vi "FEMC_TCP.vi"() -> ()   [LabVIEW 2017]
panel:
  in  "i-vクラスタ 2":T1={"start(mV)"=-1.0, "stop(mV)"=1.0, "step(mV)"=0.1, "file_name"="", "IF OFF/ON"=FALSE, "SAVE OFF/ON"=FALSE, "frq(GHz)"=8.0, "avg"=1, "Sweep回数 "=0, "VminfromSS"=0.15, "測定モード"=0, "V　opt"=2} {"測定モード" items=["電圧スイープ", "毎回HOT/COLD"]; "Sweep回数" items=["一回のみ", "Hot/Cold_auto", "Hot/Cold manual"]}
  out "GET_SIS_C 2":dbl=14.5172119140625
  out "GET_SIS_V 2":dbl=1.92230224609375
  in  "Control":T2={"GPIB_ATT"="28", "6501Dev#"=1, "GPIB_SP"="18", "GPIB_PM"="13", "GPIB_DSA"="11", "GPIB_DMM (TPD)"="23", "MPI COM"="COM5", "mortor設定"=[{"Axis"=0, "ID"=0, "HIspeed"=200.0, "LOspeed"=100.0, "ACCEL(ms)"=100.0, "Sratio"=50.0, "フリーラン\n"=FALSE, "文字列"="DSB HOT/COLD"}, {"Axis"=1, "ID"=0, "HIspeed"=4.0, "LOspeed"=4.0, "ACCEL(ms)"=100.0, "Sratio"=50.0, "フリーラン\n"=TRUE, "文字列"="SubMM Att"}, {"Axis"=0, "ID"=0, "HIspeed"=200.0, "LOspeed"=100.0, "ACCEL(ms)"=100.0, "Sratio"=50.0, "フリーラン\n"=FALSE, "文字列"="MPI Port1"}, {"Axis"=1, "ID"=0, "HIspeed"=200.0, "LOspeed"=100.0, "ACCEL(ms)"=100.0, "Sratio"=50.0, "フリーラン\n"=FALSE, "文字列"="MPI Port2"}, {"Axis"=1, "ID"=0, "HIspeed"=200.0, "LOspeed"=100.0, "ACCEL(ms)"=100.0, "Sratio"=50.0, "フリーラン\n"=TRUE, "文字列"="gainComp"}], "DATAパス"=path "C:/data/バランスドミクサ/150115/WCA_setmix_2", "mixer param file "=path "C:/data/バランスドミクサ/150115/mixparam_150115_balanced_Tmin_VSS1p5.csv", "comment"="150115_balanced_WCA_2", "Carteidge SN"="balanced150115", "Th"=297.0, "Tc"=83.26, "Set_SIS_volt"=2.1, "Offset"=0.0, "control"=0, "FreqLO"=799.0, "Set_Mag_Cur"=0.0, "MPI offset(mm)"=23.203, "HOT/COLD"=0} {"HOT/COLD" items=["DSB", "SBR (Cart.)"]; "control" items=["CLOSE LOOP", "OPEN LOOP", "Not Control"]}
  in  "i-vクラスタ":T1={"start(mV)"=-1.0, "stop(mV)"=1.0, "step(mV)"=0.1, "file_name"="", "IF OFF/ON"=FALSE, "SAVE OFF/ON"=FALSE, "frq(GHz)"=8.0, "avg"=1, "Sweep回数 "=0, "VminfromSS"=0.15, "測定モード"=0, "V　opt"=2} {"測定モード" items=["電圧スイープ", "毎回HOT/COLD"]; "Sweep回数" items=["一回のみ", "Hot/Cold_auto", "Hot/Cold manual"]}
  in  "demag":T3={"Start(mA)"=100.0, "Time(ms)"=200.0, "step"=1.0}
  in  "読み取りタイムアウト":i32=100
  in  "読み取りバイト数":i32=512
  in  "接続入力待ち（ms）":i32=10000
  out "接続回数":i32
  out "リモートポート":i16
  out "リモートアドレス":string
  out "接続中":bool
  out "GET_AMC":T4={"AMC_A_DRAIN_V"=3.5023499, "AMC_A_DRAIN_C"=53.95508, "AMC_A_GATE_V"=-0.47195435, "AMC_B_DRAIN_V"=4.3559265, "AMC_B_DRAIN_C"=314.81934, "AMC_B_GATE_V"=-0.49163818, "AMC_E_DRAIN_V"=3.9920044, "AMC_E_DRAIN_C"=338.2721, "AMC_E_GATE_V"=-0.24505615, "AMC_3V_SUPPLY_V"=-13.493347, "AMC_5V_MON"=5.223694, "AMC_MULT_D_V"=0.0}
  out "GET_PLL":T5={"PLL_ASSY_T"=35.217285, "PLL_REF_TOT_P"=-2.1250916, "PLL_IF_TOT_P"=-4.8457336, "PLL_CORR_V"=-0.14390425, "PLL_LOCK_V"=5.097532, "PLL_5V_SUPPLY_V"=18.560791, "Temp_TF"=TRUE, "PLL Ref Pwr_TF"=TRUE, "IF Pwr_TF"=TRUE, "PLL Corr_TF"=TRUE, "PLL Lock V_TF"=TRUE, "PLL Nominal_TF"=TRUE}
  out "GET_PA":T6={"PA_A_DRAIN_V"=2.3698425, "PA_A_DRAIN_C"=178.28369, "PA_A_GATE_V"=-0.3868103, "PA_B_DRAIN_V"=0.010070801, "PA_B_DRAIN_C"=5.996704, "PA_B_GATE_V"=-0.390625, "PA_3V_SUPPLY_V"=2.991333, "PA_5V_MON"=5.23407}
  out "SET_PA_VG":dbl
  out "SET_PA_VD":dbl
  out "GET_SIS_C":dbl=14.5172119140625
  out "GET_SIS_V":dbl=1.92230224609375
  out "SET_SIS_V":dbl=2.0
  in  "CLNA_SET":T7={"CLNA State"=1, "SET POL0 LNA1 STAGE1 DRAIN V"=1.2, "SET POL0 LNA1 STAGE1 DRAIN C"=14.0, "SET POL0 LNA1 STAGE2 DRAIN V"=0.0, "SET POL0 LNA1 STAGE2 DRAIN C"=0.0, "SET POL0 LNA1 STAGE3 DRAIN V"=0.0, "SET POL0 LNA1 STAGE3 DRAIN C"=0.0} {"SET POL0 LNA1 STAGE3 DRAIN C" min=0 max=20 step=0.01 format="%.2f"; "SET POL0 LNA1 STAGE3 DRAIN V" min=0 max=3 step=0.01 format="%.2f"; "SET POL0 LNA1 STAGE2 DRAIN C" min=0 max=20 step=0.01 format="%.2f"; "SET POL0 LNA1 STAGE2 DRAIN V" min=0 max=3 step=0.01 format="%.2f"; "SET POL0 LNA1 STAGE1 DRAIN C" min=0 max=20 step=0.01 format="%.2f"; "SET POL0 LNA1 STAGE1 DRAIN V" min=0 max=3 step=0.01 format="%.2f"; "CLNA State" items=["Disabled", "Enabled"]}
  out "CLNA_monitor":T8={"Pol0 LNA1 S1 Drain V [V]"=1.2019653, "Pol0 LNA1 S1 Drain C [mA]"=14.073029, "Pol0 LNA1 S1 Gate V [V]"=0.5575104, "Pol0 LNA1 S2 Drain V [V]"=0.0029144287, "Pol0 LNA1 S2 Drain C [mA]"=0.00076293945, "Pol0 LNA1 S2 Gate V [V]"=4.940506, "Pol0 LNA1 S3 Drain V [V]"=0.0027313232, "Pol0 LNA1 S3 Drain C [mA]"=0.025024414, "Pol0 LNA1 S3 Gate V [V]"=4.9404755, "Pol0 LNA1 State"=enum."Enabled"} {"Pol0 LNA1 S3 Gate V [V]" format="%.2f"; "Pol0 LNA1 S3 Drain C [mA]" format="%.2f"; "Pol0 LNA1 S3 Drain V [V]" format="%.2f"; "Pol0 LNA1 S2 Gate V [V]" format="%.2f"; "Pol0 LNA1 S2 Drain C [mA]" format="%.2f"; "Pol0 LNA1 S2 Drain V [V]" format="%.2f"; "Pol0 LNA1 S1 Gate V [V]" format="%.2f"; "Pol0 LNA1 S1 Drain C [mA]" format="%.2f"; "Pol0 LNA1 S1 Drain V [V]" format="%.2f"}
  in  "SIScontrol":u16(ring) items=["CLOSE LOOP", "OPEN LOOP", "Not Control"]
  out "option":string
  in  "Bias_LO_equip":T9={"Node address"=19, "CAN Interface"="CAN0", "Cartridge band"=8, "Slave Node in"={"Address"=19, "Serial Number"=[16, 121, 69, 76, 1, 8, 0, -31]}, "ObjHandle out"=20, "POL"=0, "sb"=1, "GPIB_SM (SIS S,V)"="24", "GPIB_DMM (SIS I)"="22", "GPIB_SM (MAG I) "="25", "GPIB_SG(LO)"="19", "GPIB_PW (PAMP) "="6", "GPIB_TMP1(8ch)"="12", "GPIB_TMP2(2ch)  "="13", "WCA_avg"=10, "Rsen"=10.0, "BiasModule"=1, "LOModule "=2, "WCA_LO_FREQ_SET"={"YTO Low freq. [GHz]"=14.65, "YTO High freq. [GHz]"=17.5, "Kvco"=1, "Lock Pol."=0, "SET LO FREQ"=88.77778, "Multiplier"=6.0, "YTO (HEX)"=210, "YTO ( FREQ)"=14.796153, "NULL PLL INTEGRATOR"=TRUE}, "Res for"=0} {"Res for" items=["none", "series res", "parallel res"]; "WCA_LO_FREQ_SET"."YTO ( FREQ)" min=25 max=150 step=0.0001 format="%.3f"; "WCA_LO_FREQ_SET"."Multiplier" min=3 max=6 step=3; "WCA_LO_FREQ_SET"."SET LO FREQ" min=25 max=150 step=0.0001 format="%.3f"; "WCA_LO_FREQ_SET"."Lock Pol." items=["Lower", "Upper"]; "WCA_LO_FREQ_SET"."Kvco" items=["7.5MHz/V", "15MHz/V"]; "WCA_LO_FREQ_SET"."YTO High freq. [GHz]" format="%.3f"; "WCA_LO_FREQ_SET"."YTO Low freq. [GHz]" format="%.3f"; "BiasModule" items=["B10Lab Bias"=0, "WCA BiasModule"=1, "none"=99]; "Slave Node in"."Serial Number" format="%.0x"; "Slave Node in"."Address" format="%.0x"; "Cartridge band" max=10 step=1; "Node address" format="%.0x"}
  out "send message":string
  in  "exit":bool=TRUE caption="停止"
  in  "stop":bool caption="停止"
  out "command:":string caption="command"
  out "c ID":refnum<k5> caption="接続ID"
  in  "Port":u16=7568 caption="サーバーポート"
  # "Vd [V]"
  # "Id [mA]"
  # "Vg [V]"
  # "AMC A"
  # "AMC B"
  # "AMC E"
  # "-3V/5V Supply"
  # "Vd [V]"
  # "Id [mA]"
  # "Vg [V]"
  # "PA A"
  # "PA B"
  # "Vd [V]"
  # "Id [mA]"
  # "Stage 1"
  # "Stage 2"
  # "Stage 3"
  # "CLNA State."
  # "Vd [V]"
  # "Id [mA]"
  # "Vg [V]"
  # "Stage 1"
  # "Stage 2"
  # "Stage 3"
  # "LO freq. [GHz]"
  # "YTO LOW\n/High Freq."
  # "ZERO Intgrtr"
  # "Node Address"
  # "Serial Number"
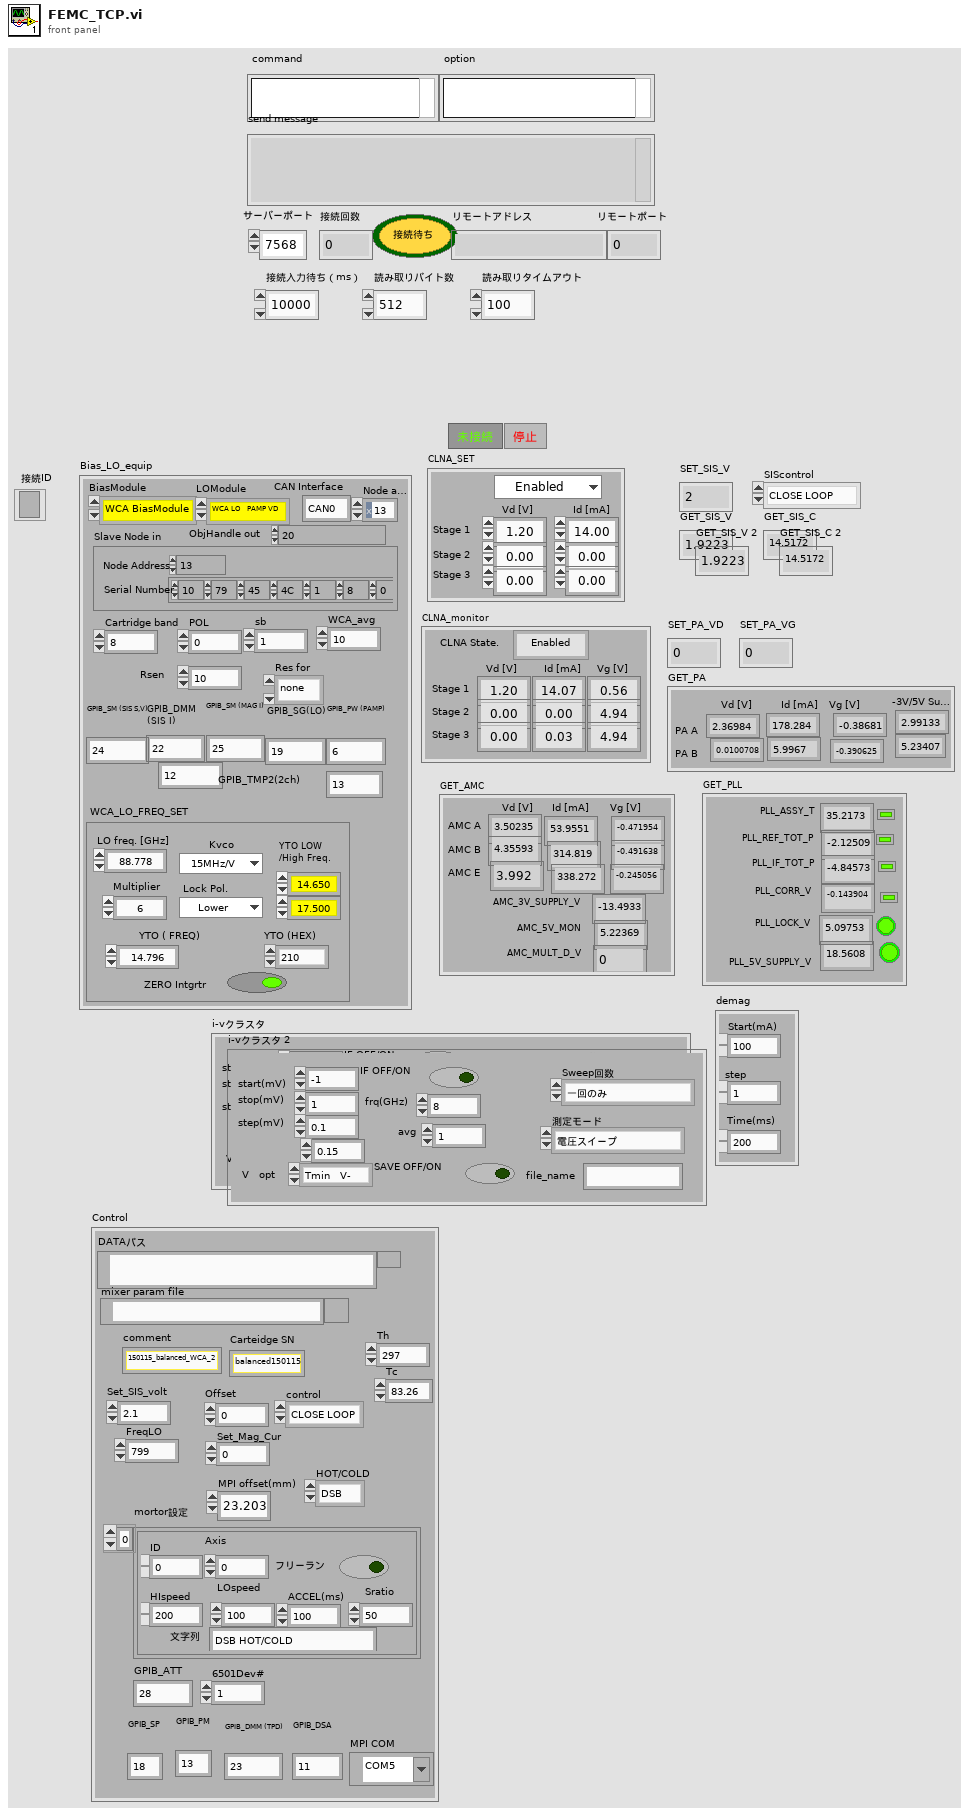
[diagram p1: front panel]
types:
  T1 = cluster{"start(mV)":dbl, "stop(mV)":dbl, "step(mV)":dbl, "file_name":string, "IF OFF/ON":bool, "SAVE OFF/ON":bool, "frq(GHz)":dbl, "avg":i32, "Sweep回数 ":u16, "VminfromSS":dbl, "測定モード":u16, "V　opt":u16}
  T2 = cluster{"GPIB_ATT":string, "6501Dev#":i16, "GPIB_SP":string, "GPIB_PM":string, "GPIB_DSA":string, "GPIB_DMM (TPD)":string, "MPI COM":refnum<visa-resource-name>, "mortor設定":cluster{"Axis":i16, "ID":i16, "HIspeed":dbl, "LOspeed":dbl, "ACCEL(ms)":dbl, "Sratio":dbl, "フリーラン\n":bool, "文字列":string}[], "DATAパス":path, "mixer param file ":path, "comment":string, "Carteidge SN":string, "Th":dbl, "Tc":dbl, "Set_SIS_volt":dbl, "Offset":dbl, "control":u16, "FreqLO":dbl, "Set_Mag_Cur":dbl, "MPI offset(mm)":dbl, "HOT/COLD":u16}
  T3 = cluster{"Start(mA)":dbl, "Time(ms)":dbl, "step":dbl}
  T4 = cluster{"AMC_A_DRAIN_V":sgl, "AMC_A_DRAIN_C":sgl, "AMC_A_GATE_V":sgl, "AMC_B_DRAIN_V":sgl, "AMC_B_DRAIN_C":sgl, "AMC_B_GATE_V":sgl, "AMC_E_DRAIN_V":sgl, "AMC_E_DRAIN_C":sgl, "AMC_E_GATE_V":sgl, "AMC_3V_SUPPLY_V":sgl, "AMC_5V_MON":sgl, "AMC_MULT_D_V":sgl}
  T5 = cluster{"PLL_ASSY_T":sgl, "PLL_REF_TOT_P":sgl, "PLL_IF_TOT_P":sgl, "PLL_CORR_V":sgl, "PLL_LOCK_V":sgl, "PLL_5V_SUPPLY_V":sgl, "Temp_TF":bool, "PLL Ref Pwr_TF":bool, "IF Pwr_TF":bool, "PLL Corr_TF":bool, "PLL Lock V_TF":bool, "PLL Nominal_TF":bool}
  T6 = cluster{"PA_A_DRAIN_V":sgl, "PA_A_DRAIN_C":sgl, "PA_A_GATE_V":sgl, "PA_B_DRAIN_V":sgl, "PA_B_DRAIN_C":sgl, "PA_B_GATE_V":sgl, "PA_3V_SUPPLY_V":sgl, "PA_5V_MON":sgl}
  T7 = cluster{"CLNA State":u8, "SET POL0 LNA1 STAGE1 DRAIN V":sgl, "SET POL0 LNA1 STAGE1 DRAIN C":sgl, "SET POL0 LNA1 STAGE2 DRAIN V":sgl, "SET POL0 LNA1 STAGE2 DRAIN C":sgl, "SET POL0 LNA1 STAGE3 DRAIN V":sgl, "SET POL0 LNA1 STAGE3 DRAIN C":sgl}
  T8 = cluster{"Pol0 LNA1 S1 Drain V [V]":sgl, "Pol0 LNA1 S1 Drain C [mA]":sgl, "Pol0 LNA1 S1 Gate V [V]":sgl, "Pol0 LNA1 S2 Drain V [V]":sgl, "Pol0 LNA1 S2 Drain C [mA]":sgl, "Pol0 LNA1 S2 Gate V [V]":sgl, "Pol0 LNA1 S3 Drain V [V]":sgl, "Pol0 LNA1 S3 Drain C [mA]":sgl, "Pol0 LNA1 S3 Gate V [V]":sgl, "Pol0 LNA1 State":enum16{"Disabled", "Enabled"}}
  T9 = cluster{"Node address":u16, "CAN Interface":string, "Cartridge band":u32, "Slave Node in":cluster{"Address":i16, "Serial Number":i8[]}, "ObjHandle out":u32, "POL":u32, "sb":u32, "GPIB_SM (SIS S,V)":string, "GPIB_DMM (SIS I)":string, "GPIB_SM (MAG I) ":string, "GPIB_SG(LO)":string, "GPIB_PW (PAMP) ":string, "GPIB_TMP1(8ch)":string, "GPIB_TMP2(2ch)  ":string, "WCA_avg":i32, "Rsen":dbl, "BiasModule":u16, "LOModule ":u16, "WCA_LO_FREQ_SET":cluster{"YTO Low freq. [GHz]":sgl, "YTO High freq. [GHz]":sgl, "Kvco":u16, "Lock Pol.":u16, "SET LO FREQ":sgl, "Multiplier":sgl, "YTO (HEX)":u16, "YTO ( FREQ)":sgl, "NULL PLL INTEGRATOR":bool}, "Res for":u16}
  T10 = cluster{"Node address":u16, "CAN Interface":string, "Cartridge band":u32, "Slave Node in":cluster{"Address":i16, "Serial Number":i8[]}, "ObjHandle out":u32, "POL":u32, "sb":u32, "GPIB_SM (SIS S,V)":string, "GPIB_DMM (SIS I)":string, "GPIB_SM (MAG I) ":string, "GPIB_SG(LO)":string, "GPIB_PW (PAMP) ":string, "GPIB_TMP1(8ch)":string, "GPIB_TMP2(2ch)  ":string, "WCA_avg":i32, "Rsen":dbl, "BiasModule":u16, "LOModule ":u16, "WCA_LO_FREQ_SET":cluster{"YTO Low freq. [GHz]":sgl, "YTO High freq. [GHz]":sgl, "Kvco":u16, "Lock Pol.":u16, "SET LO FREQ":sgl, "Multiplier":sgl, "YTO (HEX)":u16, "YTO coarse( FREQ)":sgl, "NULL PLL INTEGRATOR":bool}, "Res for":u16}
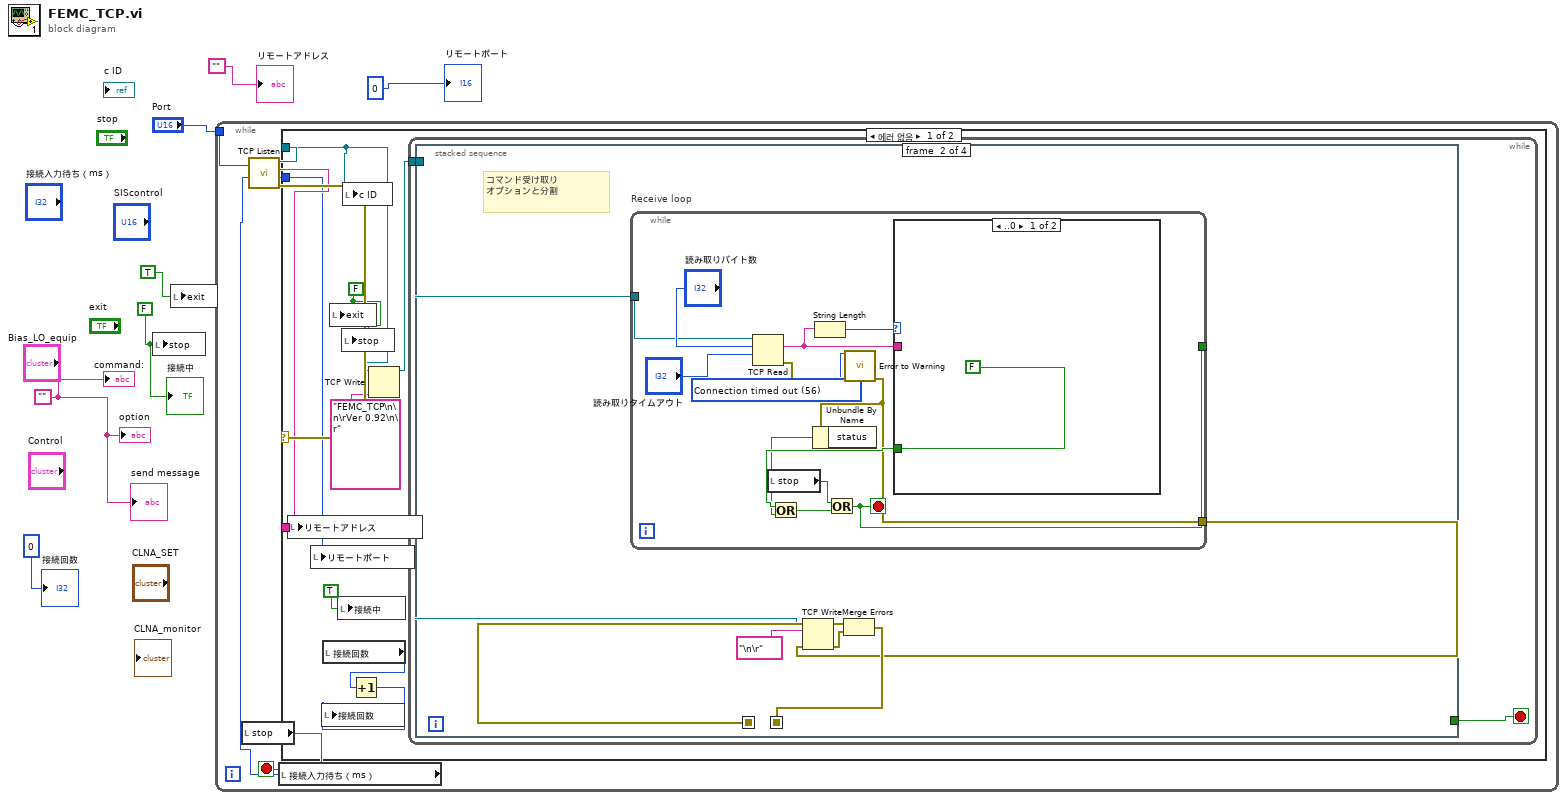
[diagram p0: block diagram]
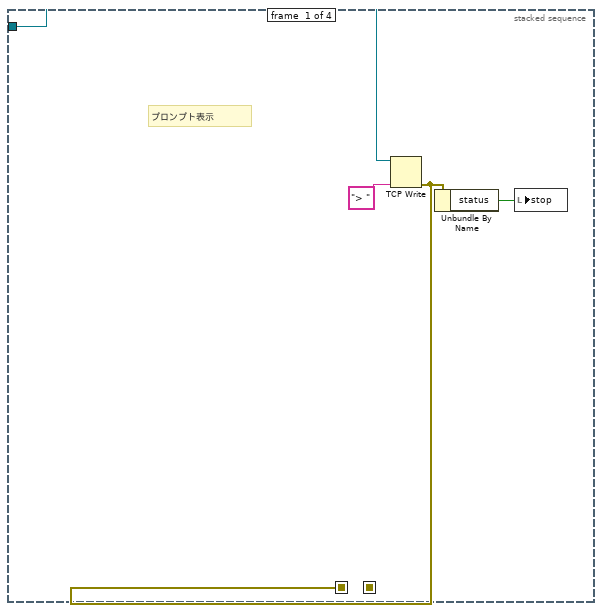
[diagram p2: hidden frame]
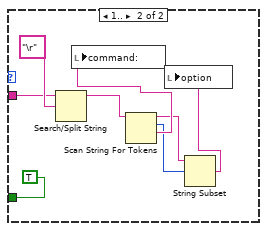
[diagram p3: hidden frame]
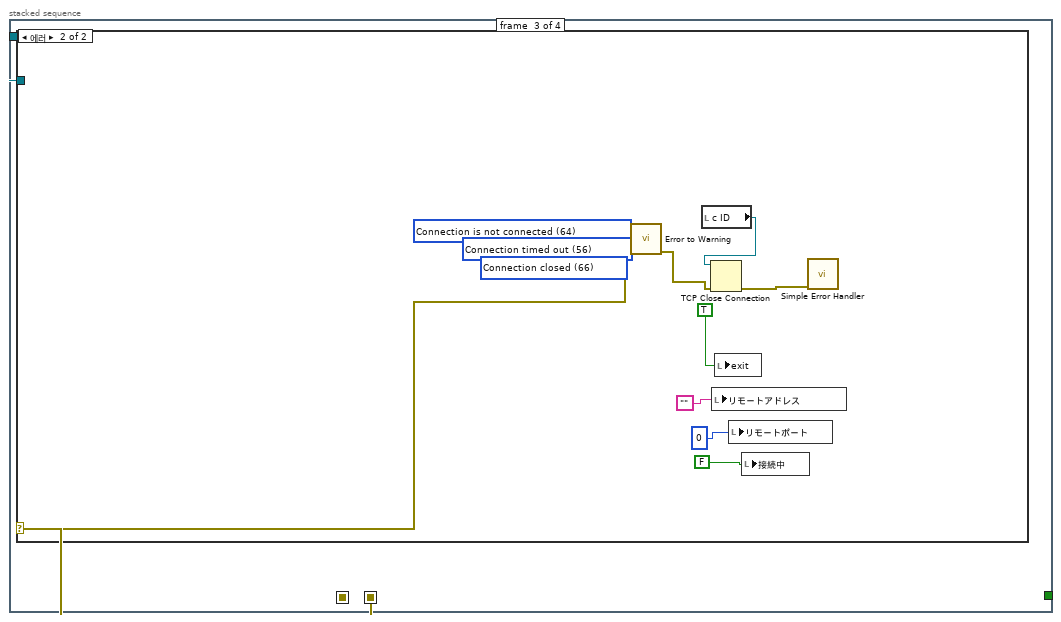
[diagram p4: hidden frame]
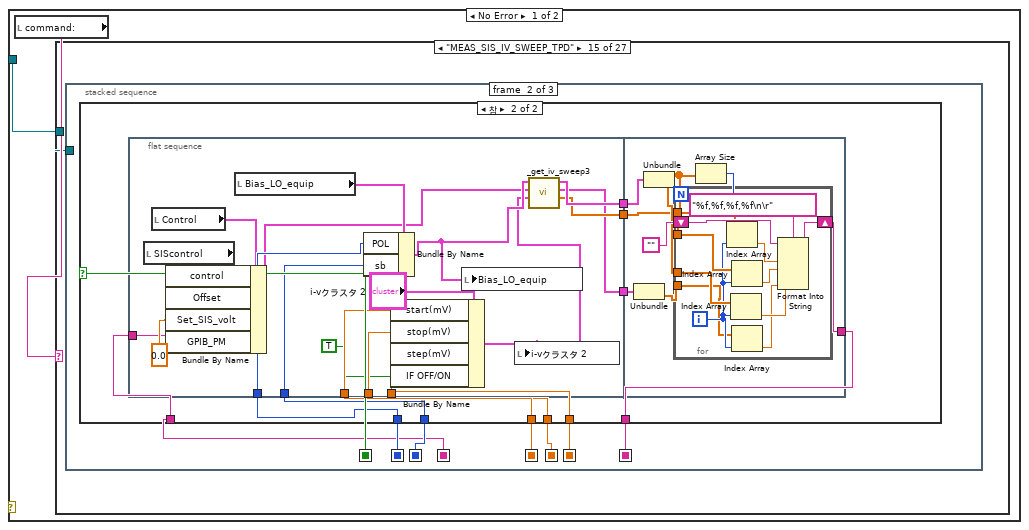
[diagram p5: hidden frame]
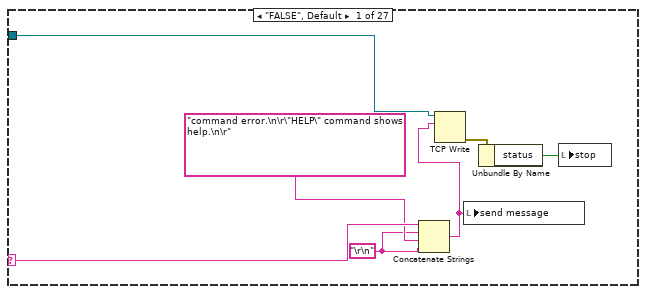
[diagram p6: hidden frame]
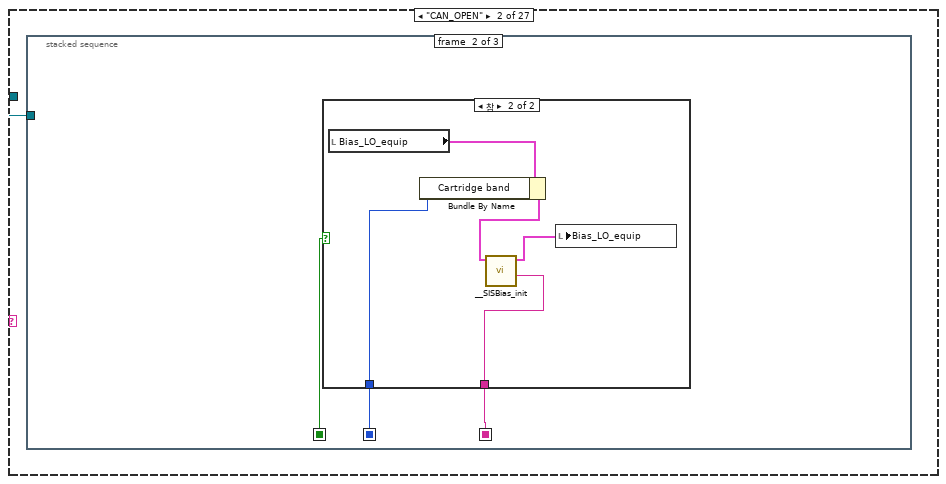
[diagram p7: hidden frame]
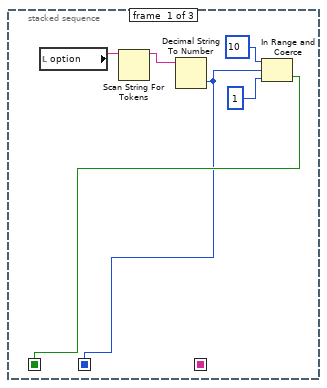
[diagram p8: hidden frame]
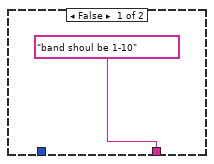
[diagram p9: hidden frame]
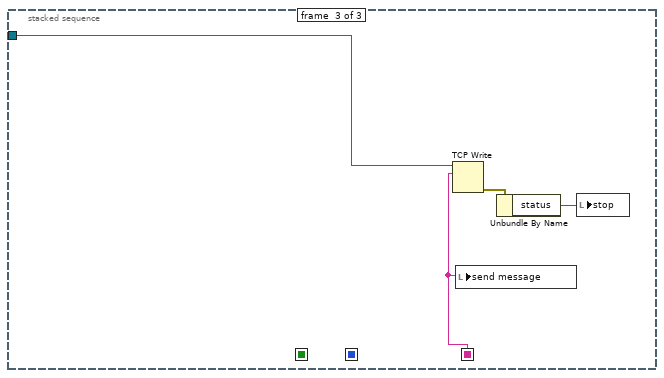
[diagram p10: hidden frame]
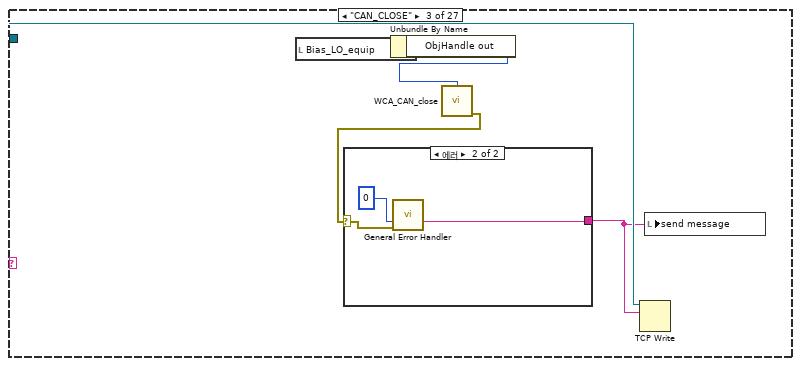
[diagram p11: hidden frame]
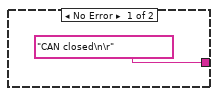
[diagram p12: hidden frame]
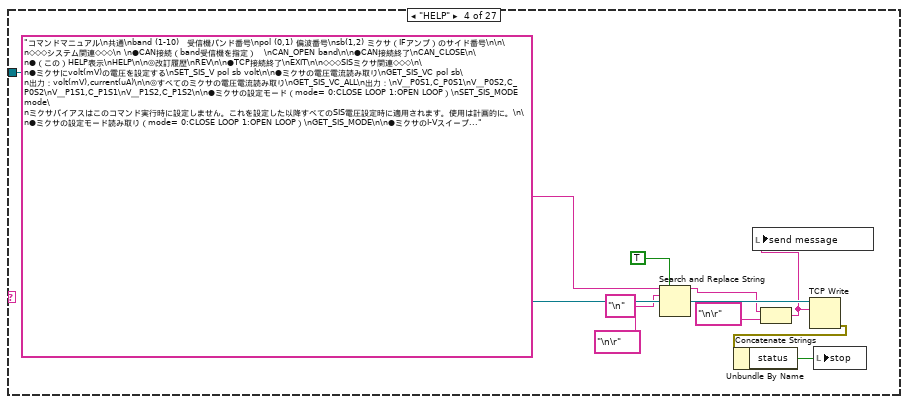
[diagram p13: hidden frame]
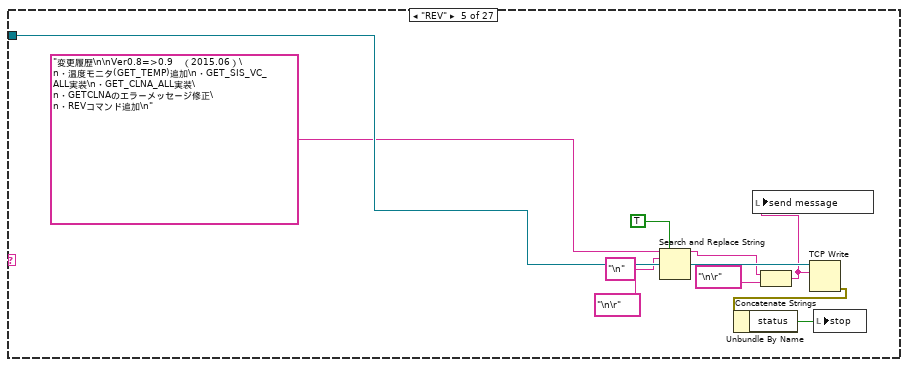
[diagram p14: hidden frame]
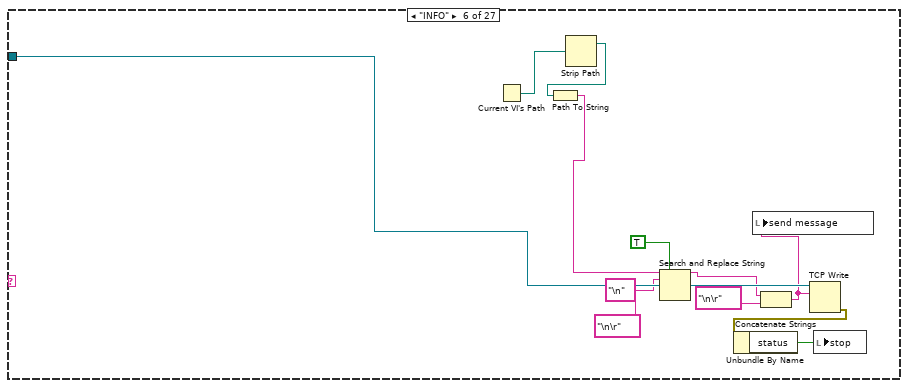
[diagram p15: hidden frame]
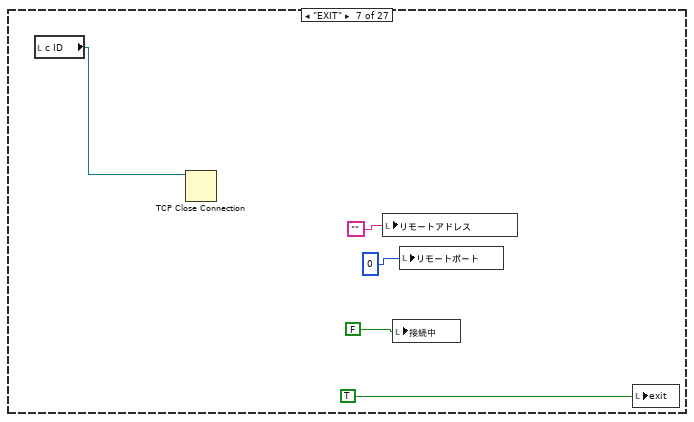
[diagram p16: hidden frame]
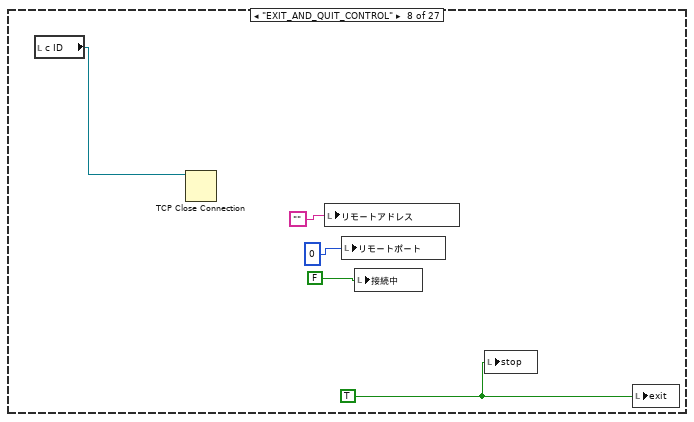
[diagram p17: hidden frame]
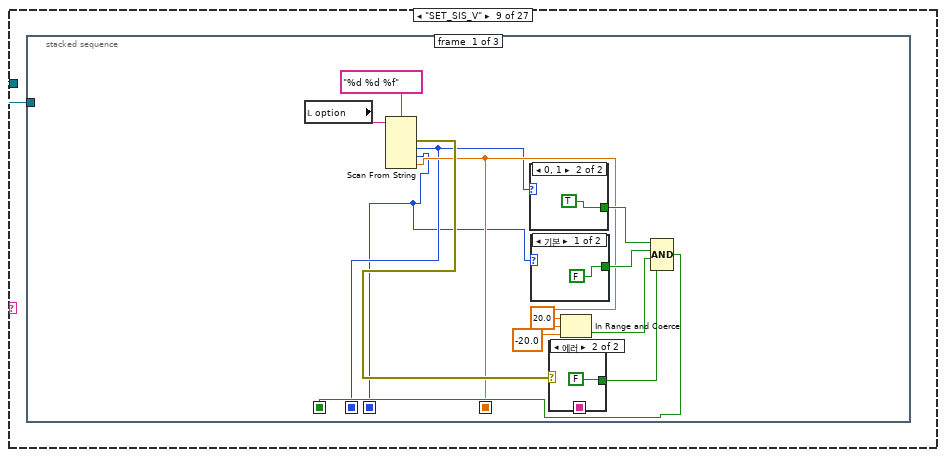
[diagram p18: hidden frame]
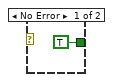
[diagram p19: hidden frame]
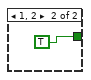
[diagram p20: hidden frame]
diagram:
  w1 = ""
  w5 = FALSE
  n1 = local write "stop"(w5) -> ()
  n2 = local write "exit"(TRUE) -> ()
  n3 = while {
    tunnel: "Port" -> [w14]
    stop <- w13 stop-if-true
    n4 = local read "stop"() -> (w13:bool)
    n5 = local read "接続入力待ち（ms）"() -> (w8:i32)
    n6 = call <vilib>:"TCP Listen.vi"("timeout ms (wait forever: -1)"=w8, "port"=w14) -> ("error out"=w12:errorcluster, "remote port"=w9:u16, "remote address"=w10:string, "connection ID"=w11:refnum<k5>)  [unwired: 5 in, 1 out]
    n7 = case shown="에러 없음" w12 {
      tunnel: w11 -> [w22 _]
      tunnel: w10 -> [w19 _]
      tunnel: w9 -> [w18 _]
      frame No Error {
        w20 = FALSE
        n8 = local write "リモートアドレス"(w19) -> ()
        n9 = local write "リモートポート"(w18) -> ()
        n10 = local read "接続回数"() -> (w16:i32)
        n11 = local write "exit"(w20) -> ()
        n12 = local write "接続中"(TRUE) -> ()
        n13 = local write "stop"(w20) -> ()
        n14 = local write "c ID"(w22) -> ()
        n15 = Increment(x=w16) -> (x+1=w15:i32)
        n16 = local write "接続回数"(w15) -> ()
        n17 = TCP Write(connection ID=w22, data in="FEMC_TCP\n\n\rVer 0.92\n\r") -> (connection ID out=w21:refnum<k5>)  [unwired: 2 in, 2 out]
        n18 = while {
          tunnel: w21 -> [w24]
          stop <- w25 stop-if-true
          n19 = stacked-sequence {
            seq-local: [w27 _ _ _] -> [_ w35 _ _]
            seq-local: [_ w34 _ _] -> [_ _ w59 _]
            tunnel: w24 -> [w29 w30 w58 _]
            tunnel: [_ _ _ w1048] -> w25
            frame #0 {
              # "プロンプト表示"
              n20 = TCP Write(connection ID=w29, data in="> ") -> (error out=w27:errorcluster)  [unwired: 2 in, 2 out]
              n21 = Unbundle By Name(w27) -> ("status"=w28:bool)
              n22 = local write "stop"(w28) -> ()
            }
            frame #1 {
              # "コマンド受け取り\nオプションと分割"
              n23 = while "Receive loop" {
                tunnel: [w45] -> _
                tunnel: [w39] -> w31
                tunnel: w30 -> [w46]
                stop <- w45 stop-if-true
                w40 = 56 items=["No Error", "Argument Error", "Memory Full", "Out of Zone", "End of File", "File Already Open", "Generic File IO Error", "File Not Found", "File Permission Error", "Disk Full", "Duplicate Path", "Too Many Files Open", "Not Enabled", "Resource File Not Found", "Cannot Add Resource", "Resource Not Found", "Image Not Found", "Image Memory Error", "Pen Does Not Exist", "Config Bad Type", "Config Token Not Found", "Config Parse Error", "Config Memory Error", "Bad External Code Format", "Bad External Code Offset", "External Code Not Present", "Null Window", "Destroy Window Mixup", "Null Menu", "Print Aborted", "Bad Print Record", "Print Driver Error", "Windows Error During Print", "Memory Error During Print", "Print Dialog Error", "Generic Print Error", "Invalid Device Refnum", "Device Not Found", "Device Parameter Error", "Device Unit Error", "Can't Open Device", "Device Call Aborted", "Generic Error", "Cancelled By User", "Object ID Too Low", "Object ID Too High", "Object Not In Heap", "Unknown Heap", "Bad DefProc ID", "DefProc Not In Table", "Message Out Of Range", "Null Method", "Unknown Message", "Manager Call Not Supported", "Bad address", "Connection In progress", "Connection timed out", "Connection is already in progress", "Network attribute not supported", "Network error", "Address in use", "System out of memory", "Connection aborted", "Connection refused", "Connection is not connected", "Connection is already connected", "Connection closed", "Initialize error (interapplication manager)", "Bad occurrence", "Wait on unbound occurrence handler", "Occurrence queue overflow", "Bad path", "Semaphore not signaled", "Unrecognized type (interapplication manager)"] ("1st Error to Convert")
                n24 = TCP Read(connection ID=w46, bytes to read="読み取りバイト数", 9:"読み取りタイムアウト") -> (data out=w44:string, error out=w41:errorcluster)  [unwired: 2 in, 1 out]
                n25 = local read "stop"() -> (w37:bool)
                n26 = String Length(string=w44) -> (length=w48:i32)
                n27 = call <vilib>:"Error to Warning.vi"("1st Error to Convert"=w40, "error in"=w41) -> ("warning out"=w39:errorcluster)  [unwired: 13 in]
                n28 = Unbundle By Name(w39) -> ("status"=w38:bool)
                n29 = case shown="..0" w48 {
                  tunnel: w44 -> [_ w55]
                  tunnel: [FALSE TRUE] -> w43
                  frame ..0 {
                  }
                  frame 1.. {
                    n30 = Search/Split String(string=w55, search string/char (-)="\r") -> (substring before match=w54:string)  [unwired: 1 in, 2 out]
                    n31 = Scan String For Tokens(9:w54) -> (1:w53:string, 2:w51:i32, 3:w52:string)  [unwired: 5 in, 1 out]
                    n32 = local write "command:"(w53) -> ()
                    n33 = String Subset(string=w52, offset (0)=w51) -> (substring=w50:string)  [unwired: 1 in]
                    n34 = local write "option"(w50) -> ()
                  }
                }
                n35 = Or(x=w43, y=w38) -> (x .or. y?=w36:bool)
                n36 = Or(x=w37, y=w36) -> (x .or. y?=w45:bool)
              }
              n37 = TCP Write(connection ID=w30, data in="\n\r", error in (no error)=w31) -> (error out=w32:errorcluster)  [unwired: 1 in, 2 out]
              n38 = Merge Errors(w35, w32) -> (w34:errorcluster)
            }
            frame #2 {
              n39 = case shown="에러" w59 {
                selector: w59 -> [_ w1041]
                tunnel: w58 -> [w61 _]
                frame No Error {
                  n40 = local read "command:"() -> (w60:string)
                  n41 = case shown="\"MEAS_SIS_IV_SWEEP_TPD\"" w60 {
                    selector: w60 -> [w65 _ _ _ _ _ _ _ _ _ _ _ _ _ _ _ _ _ _ _ _ _ _ _ _ _ _]
                    tunnel: w61 -> [w66 w69 w90 w105 w115 w127 _ _ w140 w183 w222 w250 w274 w283 w363 w454 w551 w605 w648 w691 w727 w760 w816 w858 w900 w950 w1009]
                    frame "FALSE", Default {
                      w63 = "\r\n"
                      n42 = Concatenate Strings(w65, w63, "command error.\n\r\"HELP\" command shows  help.\n\r", w63) -> (w62:string)
                      n43 = TCP Write(connection ID=w66, data in=w62) -> (error out=w67:errorcluster)  [unwired: 2 in, 2 out]
                      n44 = local write "send message"(w62) -> ()
                      n45 = Unbundle By Name(w67) -> ("status"=w68:bool)
                      n46 = local write "stop"(w68) -> ()
                    }
                    frame "CAN_OPEN" {
                      n47 = stacked-sequence {
                        seq-local: [w71 _ _] -> [_ w78 _]
                        seq-local: [w70 _ _] -> [_ w77 _]
                        seq-local: [_ w76 _] -> [_ _ w85]
                        tunnel: w69 -> [_ _ w86]
                        frame #0 {
                          n48 = local read "option"() -> (w75:string)
                          n49 = Scan String For Tokens(9:w75) -> (3:w74:string)  [unwired: 5 in, 3 out]
                          n50 = Decimal String To Number(string=w74) -> (number=w70:i32)  [unwired: 2 in, 1 out]
                          n51 = In Range and Coerce(upper limit=10, x=w70, lower limit=1) -> (In Range?=w71:bool)  [unwired: 1 out]
                        }
                        frame #1 {
                          n52 = case shown="참" w78 {
                            tunnel: w77 -> [_ w83]
                            tunnel: ["band shoul be 1-10" w80] -> w76
                            frame False {
                            }
                            frame True {
                              n53 = local read "Bias_LO_equip"() -> (w84:T9)
                              n54 = Bundle By Name(cluster=w84, "Cartridge band"=w83) -> (w82:T9)
                              n55 = call "__SISBias_init.vi"("Bias_LO_equip"=w82) -> ("Detected CAN Nodes."=w80:string, "Bias_LO_equip 2"=w81:T10)  [unwired: 4 in, 1 out]
                              n56 = local write "Bias_LO_equip"(w81) -> ()
                            }
                          }
                        }
                        frame #2 {
                          n57 = TCP Write(connection ID=w86, data in=w85) -> (error out=w87:errorcluster)  [unwired: 2 in, 2 out]
                          n58 = local write "send message"(w85) -> ()
                          n59 = Unbundle By Name(w87) -> ("status"=w88:bool)
                          n60 = local write "stop"(w88) -> ()
                        }
                      }
                    }
                    frame "CAN_CLOSE" {
                      n61 = local read "Bias_LO_equip"() -> (w93:T9)
                      n62 = Unbundle By Name(w93) -> ("ObjHandle out"=w92:u32)
                      n63 = call "WCA_CAN_close.vi"("ObjHandle in"=w92) -> ("error out"=w91:errorcluster)  [unwired: 14 in]
                      n64 = case shown="에러" w91 {
                        selector: w91 -> [_ w97]
                        tunnel: ["CAN closed\n\r" w96] -> w89
                        frame No Error {
                        }
                        frame Error {
                          n65 = call <vilib>:"General Error Handler.vi"("type of dialog (OK msg:1)"=0, "error in (no error)"=w97) -> ("message"=w96:string)  [unwired: 9 in, 4 out]
                        }
                      }
                      n66 = TCP Write(connection ID=w90, data in=w89) -> ()  [unwired: 2 in, 3 out]
                      n67 = local write "send message"(w89) -> ()
                    }
                    frame "HELP" {
                      n68 = Search and Replace String(replace all?=TRUE, input string="コマンドマニュアル\n共通\nband (1-10)　受信機バンド番号\npol (0,1) 偏波番号\nsb(1,2) ミクサ（IFアンプ）のサイド番号\n\n\n◇◇◇システム関連◇◇◇\n \n●CAN接続（band受信機を指定）　\nCAN_OPEN band\n\n●CAN接続終了\nCAN_CLOSE\n\n●（この）HELP表示\nHELP\n\n◎改訂履歴\nREV\n\n●TCP接続終了\nEXIT\n\n◇◇◇SISミクサ関連◇◇◇\n\n●ミクサにvolt(mV)の電圧を設定する\nSET_SIS_V pol sb volt\n\n●ミクサの電圧電流読み取り\nGET_SIS_VC pol sb\n出力：volt(mV),current(uA)\n\n◎すべてのミクサの電圧電流読み取り\nGET_SIS_VC_ALL\n出力：\nV＿P0S1,C_P0S1\nV＿P0S2,C_P0S2\nV＿P1S1,C_P1S1\nV＿P1S2,C_P1S2\n\n●ミクサの設定モード（mode= 0:CLOSE LOOP 1:OPEN LOOP）\nSET_SIS_MODE mode\nミクサバイアスはこのコマンド実行時に設定しません。これを設定した以降すべてのSIS電圧設定時に適用されます。使用は計画的に。\n\n●ミクサの設定モード読み取り（mode= 0:CLOSE LOOP 1:OPEN LOOP）\nGET_SIS_MODE\n\n●ミクサのI-Vスイープ\nMEAS_SIS_IV_SWEEP pol sb start stop step\n出力：v,iの連続データ\n\n●ミクサのI-VスイープWHSFのTPDからデータ取得\nMEAS_SIS_IV_SWEEP_TPD pol sb start stop step IP_TPDnum\n\nIP_TPD_num:TPD//IPアドレス//TPD番号（1から8）\n例：TPD//192.168.11.194//1\n出力：v,iの連続データ\n\n\n◇◇◇CLNA関連◇◇◇\n\n●CLNAにVD=vd#(V),ID=id#(mA)のバイアス設定(と同時に電源ONします)\nSET_CLNA pol sb vd1 id1 vd2 id2 vg3 id3\n\n●CLNAのバイアス読み取り\nGET_CLNA pol sb\n出力：vd1(V),id1(mA),vg1(V),vd2(V),id2(mA)vg2(V),vd3(V),id3(mA)vg3(V),ENABLED(1) or DISABLED(0)\n\n●CLNAの電源OFF\nSET_CLNA_OFF pol sb\n\n◎すべてのCLNAのバイアス読み取り\nGET_CLNA_ALL \n出力：\nP0S1:vd1(V),id1(mA),vg1(V),vd2(V),id2(mA)vg2(V),vd3(V),id3(mA)vg3(V),ENABLED(1) or DISABLED(0)\nP0S2:vd1(V),id1(mA),vg1(V),vd2(V),id2(mA)vg2(V),vd3(V),id3(mA)vg3(V),ENABLED(1) or DISABLED(0)\nP1S1:vd1(V),id1(mA),vg1(V),vd2(V),id2(mA)vg2(V),vd3(V),id3(mA)vg3(V),ENABLED(1) or DISABLED(0)\nP1S2:vd1(V),id1(mA),vg1(V),vd2(V),id2(mA)vg2(V),vd3(V),id3(mA)vg3(V),ENABLED(1) or DISABLED(0)\n\n\n\n◇◇◇超伝導コイル関連◇◇◇\n\n●超伝導コイル　current(mA)設定\nSET_MAG_C pol sb current\n\n●超伝導コイル電圧電流読み取り\nGET_MAG_VC pol sb(範囲確認)\n出力：volt(V),current(mA)\n\n●超伝導コイル　消磁（demag,deflux）\nACT_DEMAG pol sb start step time\nstart(mA)からstep(mA)毎にtime(ms)で0mAになるまでDemagを行う。\n実行時設定電流は以下の通り、\n+start, 0, -start, 0,\n+(start-step), 0,-(start-step)\n, , , \n0\n\n\n\n◇◇◇WCA-LO関連◇◇◇\n\n●LO PAMPのvd(V)設定（pol=0:PA-A 1:PA-B）\nSET_PA_VD pol vd(範囲確認)\n\n●LO PAMPのvg(V)設定（pol=0:PA-A 1:PA-B）\nSET_PA_VG pol vg(範囲確認)\n\n●LO PAMPのvd(V),vg(V)読み取り（pol=0:PA-A 1:PA-B）\nGET_PA pol\n出力：vd(V),id(mA),vg(V)\n\n●WCA_LOの電源等パラメータ読み取り\nGET_WCA_LO \n出力：\nPAA VD,PAA ID,PAA Vg,\nPAB VD,PAB ID,PAB Vg,\nPA -3V,PA+5V,\nPLL_ASSY_T,PLL_REF_TOT_P,PLL_IF_TOT_P,PLL_CORR_V,PLL_LOCK_V,PLL_5V,\nAMCA VD,AMCA ID,AMCA Vg,\nAMCB VD,AMCB ID,AMCB Vg,\nAMCE VD,AMCE ID,AMCE Vg,\nAMC_3V,AMC_5V,AMC_multi\n\n\n\n◇◇◇Tempモニタ関連◇◇◇\n\n◎温度センサ読み取り\nGET_TEMP pol\n出力：4KTMP,110KTMP(15KTMP),MXRTMP\n\n\n（◎今回追加したコマンド）", search string="\n", replace string="\n\r") -> (result string=w100:string)  [unwired: 4 in, 3 out]
                      n69 = Concatenate Strings(w100, "\n\r") -> (w98:string)
                      n70 = local write "send message"(w98) -> ()
                      n71 = TCP Write(connection ID=w105, data in=w98) -> (error out=w106:errorcluster)  [unwired: 2 in, 2 out]
                      n72 = Unbundle By Name(w106) -> ("status"=w107:bool)
                      n73 = local write "stop"(w107) -> ()
                    }
                    frame "REV" {
                      n74 = Search and Replace String(replace all?=TRUE, input string="変更履歴\n\nVer0.8=>0.9　（2015.06）\n・温度モニタ(GET_TEMP)追加\n・GET_SIS_VC_ALL実装\n・GET_CLNA_ALL実装\n・GETCLNAのエラーメッセージ修正\n・REVコマンド追加\n", search string="\n", replace string="\n\r") -> (result string=w111:string)  [unwired: 4 in, 3 out]
                      n75 = Concatenate Strings(w111, "\n\r") -> (w109:string)
                      n76 = local write "send message"(w109) -> ()
                      n77 = TCP Write(connection ID=w115, data in=w109) -> (error out=w116:errorcluster)  [unwired: 2 in, 2 out]
                      n78 = Unbundle By Name(w116) -> ("status"=w117:bool)
                      n79 = local write "stop"(w117) -> ()
                    }
                    frame "INFO" {
                      n80 = Current VI's Path() -> (path=w119:path)
                      n81 = Strip Path(path=w119) -> (stripped path=w118:path)  [unwired: 1 out]
                      n82 = Path To String(path=w118) -> (string=w120:string)
                      n83 = Search and Replace String(replace all?=TRUE, input string=w120, search string="\n", replace string="\n\r") -> (result string=w123:string)  [unwired: 4 in, 3 out]
                      n84 = Concatenate Strings(w123, "\n\r") -> (w121:string)
                      n85 = local write "send message"(w121) -> ()
                      n86 = TCP Write(connection ID=w127, data in=w121) -> (error out=w128:errorcluster)  [unwired: 2 in, 2 out]
                      n87 = Unbundle By Name(w128) -> ("status"=w129:bool)
                      n88 = local write "stop"(w129) -> ()
                    }
                    frame "EXIT" {
                      n89 = local read "c ID"() -> (w133:refnum<k5>)
                      n90 = TCP Close Connection(connection ID=w133) -> ()  [unwired: 2 in, 2 out]
                      n91 = local write "リモートアドレス"("") -> ()
                      n92 = local write "接続中"(FALSE) -> ()
                      n93 = local write "リモートポート"(0) -> ()
                      n94 = local write "exit"(TRUE) -> ()
                    }
                    frame "EXIT_AND_QUIT_CONTROL" {
                      w138 = TRUE
                      n95 = local read "c ID"() -> (w139:refnum<k5>)
                      n96 = TCP Close Connection(connection ID=w139) -> ()  [unwired: 2 in, 2 out]
                      n97 = local write "リモートアドレス"("") -> ()
                      n98 = local write "リモートポート"(0) -> ()
                      n99 = local write "接続中"(FALSE) -> ()
                      n100 = local write "stop"(w138) -> ()
                      n101 = local write "exit"(w138) -> ()
                    }
                    frame "SET_SIS_V" {
                      n102 = stacked-sequence {
                        seq-local: [w144 _ _] -> [_ w164 _]
                        seq-local: [w141 _ _] -> [_ w161 _]
                        seq-local: [w143 _ _] -> [_ w160 _]
                        seq-local: [w142 _ _] -> [_ w162 _]
                        seq-local: [_ w163 _] -> [_ _ w179]
                        tunnel: w140 -> [_ _ w180]
                        frame #0 {
                          n103 = local read "option"() -> (w153:string)
                          n104 = Scan From String(format string="%d %d %f", input string=w153) -> (error out=w146:errorcluster, output 1=w142:i32, output 2=w141:i32, output 3=w143:dbl)  [unwired: 5 in, 2 out]
                          n105 = case shown="0, 1" w142 {
                            tunnel: [FALSE TRUE] -> w149
                            frame Default {
                            }
                            frame 0, 1 {
                            }
                          }
                          n106 = case shown="기본" w141 {
                            tunnel: [FALSE TRUE] -> w148
                            frame Default {
                            }
                            frame 1, 2 {
                            }
                          }
                          n107 = case shown="에러" w146 {
                            tunnel: [TRUE FALSE] -> w145
                            frame No Error {
                            }
                            frame Error {
                            }
                          }
                          n108 = In Range and Coerce(upper limit=20.0, x=w143, lower limit=-20.0) -> (In Range?=w147:bool)  [unwired: 1 out]
                          n109 = Compound Arithmetic op=AND(w149, w148, w147, w145) -> (w144:bool)
                        }
                        frame #1 {
                          n110 = case shown="참" w164 {
                            tunnel: ["command error\n\rSET_SIS_V pol(0 or 1) sb(1 or 2) V(-20 to 20) \n\r" w170] -> w163
                            tunnel: w162 -> [_ w169]
                            tunnel: w161 -> [_ w168]
                            tunnel: w160 -> [_ w166]
                            frame False {
                            }
                            frame True {
                              n111 = local read "Bias_LO_equip"() -> (w174:T9)
                              n112 = local read "SIScontrol"() -> (w172:u16)
                              n113 = Bundle By Name(cluster=w174, "POL"=w169, "sb"=w168) -> (w173:T9)
                              n114 = local write "Bias_LO_equip"(w173) -> ()
                              n115 = call "__SISbias_Set.vi"("SIS　Mode"=w172, "Offset"=0.0, "Set_V"=w166, "Bias_LO_equip"=w173) -> ("error out"=w171:errorcluster)  [unwired: 7 in]
                              n116 = case shown="에러 없음" w171 {
                                selector: w171 -> [_ w177]
                                tunnel: ["OK\n\r" w176] -> w170
                                frame No Error {
                                }
                                frame Error {
                                n117 = call <vilib>:"General Error Handler.vi"("type of dialog (OK msg:1)"=0, "error in (no error)"=w177) -> ("message"=w176:string)  [unwired: 9 in, 4 out]
                                }
                              }
                              "SET_SIS_V" <- w166
                            }
                          }
                        }
                        frame #2 {
                          n118 = TCP Write(connection ID=w180, data in=w179) -> (error out=w181:errorcluster)  [unwired: 2 in, 2 out]
                          n119 = Unbundle By Name(w181) -> ("status"=w182:bool)
                          n120 = local write "send message"(w179) -> ()
                          n121 = local write "stop"(w182) -> ()
                        }
                      }
                    }
                    frame "GET_SIS_VC" {
                      n122 = stacked-sequence {
                        seq-local: [w187 _ _] -> [_ w202 _]
                        seq-local: [w184 _ _] -> [_ w199 _]
                        seq-local: [w185 _ _] -> [_ w200 _]
                        seq-local: [_ w201 _] -> [_ _ w218]
                        tunnel: w183 -> [_ _ w219]
                        frame #0 {
                          n123 = local read "option"() -> (w192:string)
                          n124 = Scan From String(format string="%d %d", input string=w192) -> (error out=w188:errorcluster, output 1=w185:i32, output 2=w184:i32)  [unwired: 4 in, 2 out]
                          n125 = case shown="에러" w188 {
                            tunnel: [TRUE FALSE] -> w186
                            frame No Error {
                            }
                            frame Error {
                            }
                          }
                          n126 = case shown="0, 1" w185 {
                            tunnel: [FALSE TRUE] -> w190
                            frame Default {
                            }
                            frame 0, 1 {
                            }
                          }
                          n127 = case shown="기본" w184 {
                            tunnel: [FALSE TRUE] -> w189
                            frame Default {
                            }
                            frame 1, 2 {
                            }
                          }
                          n128 = Compound Arithmetic op=AND(w190, w189, w186) -> (w187:bool)
                        }
                        frame #1 {
                          n129 = case shown="참" w202 {
                            tunnel: ["command error\n\rGET_SIS_VC pol(0 or 1) sb(1 or 2)" w212] -> w201
                            tunnel: w200 -> [_ w207]
                            tunnel: w199 -> [_ w206]
                            frame False {
                            }
                            frame True {
                              n130 = local read "Bias_LO_equip"() -> (w213:T9)
                              n131 = Bundle By Name(cluster=w213, "POL"=w207, "sb"=w206) -> (w211:T9)
                              n132 = call "__SISbias_Get.vi"("Bias_LO_equip"=w211) -> ("error out"=w210:errorcluster, "Get_I(uA)"=w204:dbl, "Get_V(mV)"=w205:dbl)  [unwired: 8 in]
                              "GET_SIS_C" <- w204
                              "GET_SIS_V" <- w205
                              n133 = local write "Bias_LO_equip"(w211) -> ()
                              n134 = Format Into String(format string="%f,%f\n\r", w205, w204) -> (resulting string=w208:string)  [unwired: 2 in, 1 out]
                              n135 = case shown="에러 없음" w210 {
                                selector: w210 -> [_ w216]
                                tunnel: [w214 w215] -> w212
                                tunnel: w208 -> [w214 _]
                                frame No Error {
                                }
                                frame Error {
                                n136 = call <vilib>:"General Error Handler.vi"("type of dialog (OK msg:1)"=0, "error in (no error)"=w216) -> ("message"=w215:string)  [unwired: 9 in, 4 out]
                                }
                              }
                            }
                          }
                        }
                        frame #2 {
                          n137 = TCP Write(connection ID=w219, data in=w218) -> (error out=w220:errorcluster)  [unwired: 2 in, 2 out]
                          n138 = Unbundle By Name(w220) -> ("status"=w221:bool)
                          n139 = local write "stop"(w221) -> ()
                          n140 = local write "send message"(w218) -> ()
                        }
                      }
                    }
                    frame "GET_SIS_VC_ALL" {
                      n141 = stacked-sequence {
                        seq-local: [w223 _] -> [_ w246]
                        tunnel: w222 -> [_ w247]
                        frame #0 {
                          n142 = for {
                            N: 2 -> [_]
                            shift-right: [w226] -> w223
                            shift-left: "" -> [w227]
                            i -> [w228]
                            n143 = for {
                              N: 2 -> [_]
                              tunnel: w228 -> [w232]
                              shift-right: [w230] -> w226
                              shift-left: w227 -> [w231]
                              i -> [w234]
                              # "SBループ"
                              n144 = Increment(x=w234) -> (x+1=w233:i32)
                              n145 = local read "Bias_LO_equip"() -> (w241:T9)
                              n146 = Bundle By Name(cluster=w241, "POL"=w232, "sb"=w233) -> (w240:T9)
                              n147 = call "__SISbias_Get.vi"("Bias_LO_equip"=w240) -> ("error out"=w239:errorcluster, "Get_I(uA)"=w235:dbl, "Get_V(mV)"=w236:dbl)  [unwired: 8 in]
                              "GET_SIS_C 2" <- w235
                              "GET_SIS_V 2" <- w236
                              n148 = local write "Bias_LO_equip"(w240) -> ()
                              n149 = Format Into String(format string="%f,%f\n\r", initial string=w231, w236, w235) -> (resulting string=w237:string)  [unwired: 1 in, 1 out]
                              n150 = case shown="에러 없음" w239 {
                                selector: w239 -> [_ w244]
                                tunnel: [w242 w243] -> w230
                                tunnel: w237 -> [w242 _]
                                frame No Error {
                                }
                                frame Error {
                                n151 = call <vilib>:"General Error Handler.vi"("type of dialog (OK msg:1)"=0, "error in (no error)"=w244) -> ("message"=w243:string)  [unwired: 9 in, 4 out]
                                }
                              }
                            }
                          }
                        }
                        frame #1 {
                          n152 = TCP Write(connection ID=w247, data in=w246) -> (error out=w248:errorcluster)  [unwired: 2 in, 2 out]
                          n153 = Unbundle By Name(w248) -> ("status"=w249:bool)
                          n154 = local write "stop"(w249) -> ()
                          n155 = local write "send message"(w246) -> ()
                        }
                      }
                    }
                    frame "SET_SIS_MODE" {
                      n156 = stacked-sequence {
                        seq-local: [w253 _ _] -> [_ w264 _]
                        seq-local: [w251 _ _] -> [_ w262 _]
                        seq-local: [_ w263 _] -> [_ _ w270]
                        tunnel: w250 -> [_ _ w271]
                        frame #0 {
                          n157 = local read "option"() -> (w257:string)
                          n158 = Scan From String(format string="%d", input string=w257) -> (error out=w254:errorcluster, output 1=w251:i32)  [unwired: 3 in, 2 out]
                          n159 = case shown="에러" w254 {
                            tunnel: [TRUE FALSE] -> w252
                            frame No Error {
                            }
                            frame Error {
                            }
                          }
                          n160 = case shown="0, 1" w251 {
                            tunnel: [FALSE TRUE] -> w255
                            frame Default {
                            }
                            frame 0, 1 {
                            }
                          }
                          n161 = Compound Arithmetic op=AND(w255, w252) -> (w253:bool)
                        }
                        frame #1 {
                          n162 = case shown="참" w264 {
                            tunnel: ["command error\n\rSET_SIS_MODE model(0 or 1)" w266] -> w263
                            tunnel: w262 -> [_ w267]
                            frame False {
                            }
                            frame True {
                              n163 = local write "SIScontrol"(w267) -> ()
                              n164 = case shown="0, 기본" w267 {
                                tunnel: ["SET SIS MODE:CLOSE LOOP\n\r" "SET SIS MODE:OPEN LOOP\n\r"] -> w266
                                frame 0, Default {
                                }
                                frame 1 {
                                }
                              }
                            }
                          }
                        }
                        frame #2 {
                          n165 = local write "send message"(w270) -> ()
                          n166 = TCP Write(connection ID=w271, data in=w270) -> (error out=w272:errorcluster)  [unwired: 2 in, 2 out]
                          n167 = Unbundle By Name(w272) -> ("status"=w273:bool)
                          n168 = local write "stop"(w273) -> ()
                        }
                      }
                    }
                    frame "GET_SIS_MODE" {
                      n169 = stacked-sequence {
                        seq-local: [w275 _] -> [_ w279]
                        tunnel: w274 -> [_ w280]
                        frame #0 {
                          n170 = local read "SIScontrol"() -> (w278:u16)
                          n171 = Number To Decimal String(number=w278) -> (decimal integer string=w277:string)  [unwired: 1 in]
                          n172 = Concatenate Strings(w277, "\n\r") -> (w275:string)
                        }
                        frame #1 {
                          n173 = TCP Write(connection ID=w280, data in=w279) -> (error out=w281:errorcluster)  [unwired: 2 in, 2 out]
                          n174 = Unbundle By Name(w281) -> ("status"=w282:bool)
                          n175 = local write "stop"(w282) -> ()
                          n176 = local write "send message"(w279) -> ()
                        }
                      }
                    }
                    frame "MEAS_SIS_IV_SWEEP" {
                      n177 = stacked-sequence {
                        seq-local: [w295 _ _] -> [_ w317 _]
                        seq-local: [w292 _ _] -> [_ w314 _]
                        seq-local: [w294 _ _] -> [_ w313 _]
                        seq-local: [w293 _ _] -> [_ w315 _]
                        seq-local: [_ w316 _] -> [_ _ w359]
                        seq-local: [w285 _ _] -> [_ w312 _]
                        seq-local: [w284 _ _] -> [_ w311 _]
                        tunnel: w283 -> [_ _ w360]
                        frame #0 {
                          n178 = local read "option"() -> (w304:string)
                          n179 = Scan From String(format string="%d %d %f %f %f", input string=w304) -> (error out=w297:errorcluster, output 1=w293:i32, output 2=w292:i32, output 3=w294:dbl, output 4=w285:dbl, output 5=w284:dbl)  [unwired: 7 in, 2 out]
                          n180 = case shown="에러" w297 {
                            tunnel: [TRUE FALSE] -> w296
                            frame No Error {
                            }
                            frame Error {
                            }
                          }
                          n181 = case shown="0, 1" w293 {
                            tunnel: [FALSE TRUE] -> w300
                            frame Default {
                            }
                            frame 0, 1 {
                            }
                          }
                          n182 = case shown="기본" w292 {
                            tunnel: [FALSE TRUE] -> w299
                            frame Default {
                            }
                            frame 1, 2 {
                            }
                          }
                          n183 = In Range and Coerce(upper limit=5.0, x=w284, lower limit=-5.0) -> (In Range?=w286:bool)  [unwired: 1 out]
                          n184 = In Range and Coerce(upper limit=20.0, x=w285, lower limit=-20.0) -> (In Range?=w287:bool)  [unwired: 1 out]
                          n185 = In Range and Coerce(upper limit=20.0, x=w294, lower limit=-20.0) -> (In Range?=w298:bool)  [unwired: 1 out]
                          n186 = Compound Arithmetic op=AND(w300, w299, w298, w296, w287, w286) -> (w295:bool)
                        }
                        frame #1 {
                          n187 = case shown="참" w317 {
                            tunnel: ["command error\n\rMRAS_SIS_IV_SWEEP pol(0 or 1) sb(1 or 2) start(-20 to 20) stop(-20 to 20) step(-5 to 5) \n\r" w321] -> w316
                            tunnel: w315 -> [_ w326]
                            tunnel: w314 -> [_ w325]
                            tunnel: w313 -> [_ w324]
                            tunnel: w312 -> [_ w323]
                            tunnel: w311 -> [_ w322]
                            frame False {
                            }
                            frame True {
                              n188 = flat-sequence {
                                tunnel: w326 -> [w340]
                                tunnel: w325 -> [w339]
                                tunnel: w324 -> [w338]
                                tunnel: w323 -> [w335]
                                tunnel: w322 -> [w334]
                                tunnel: [w328] -> w320
                                tunnel: [w327] -> w319
                                tunnel: [w343] -> w321
                                tunnel: w320 -> [w348]
                                tunnel: w319 -> [w342]
                                frame #0 {
                                w330 = 0.0
                                n189 = local read "SIScontrol"() -> (w331:u16)
                                n190 = local read "Control"() -> (w332:T2)
                                n191 = Bundle By Name(cluster=w332, "control"=w331, "Offset"=w330, "Set_SIS_volt"=w330) -> (w329:T2)
                                n192 = local read "Bias_LO_equip"() -> (w341:T9)
                                n193 = Bundle By Name(cluster=w341, "POL"=w340, "sb"=w339) -> (w337:T9)
                                n194 = Bundle By Name(cluster="i-vクラスタ", "start(mV)"=w338, "stop(mV)"=w335, "step(mV)"=w334) -> (w333:T1)
                                n195 = local write "Bias_LO_equip"(w337) -> ()
                                n196 = local write "i-vクラスタ"(w333) -> ()
                                n197 = call "_get_iv_sweep3.vi"("i-vクラスタ"=w333, "Control"=w329, "Bias_LO_equip"=w337) -> ("Vset"=w327:dbl[], "VIデータクラスタ"=w328:cluster{"配列":dbl[], "配列 2":dbl[]})  [unwired: 2 in, 1 out]
                                }
                                frame #1 {
                                n198 = Unbundle(w348) -> ("配列"=w345:dbl[], "配列 2"=w344:dbl[])
                                n199 = Array Size(array=w345) -> (size(s)=w347:i32)
                                n200 = for {
                                N: w347 -> [_]
                                shift-right: [w355] -> w343
                                shift-left: "" -> [w356]
                                tunnel: w345 -> [w358]
                                tunnel: w344 -> [w357]
                                tunnel: w342 -> [w352]
                                i -> [w351]
                                n201 = Index Array(array=w352, index=w351) -> (element=w353:dbl)
                                n202 = Index Array(array=w357, index=w351) -> (element=w349:dbl)
                                n203 = Index Array(array=w358, index=w351) -> (element=w350:dbl)
                                n204 = Format Into String(format string="%f,%f,%f\n\r", initial string=w356, w353, w350, w349) -> (resulting string=w355:string)  [unwired: 1 in, 1 out]
                                }
                                }
                              }
                            }
                          }
                        }
                        frame #2 {
                          n205 = TCP Write(connection ID=w360, data in=w359) -> (error out=w361:errorcluster)  [unwired: 2 in, 2 out]
                          n206 = Unbundle By Name(w361) -> ("status"=w362:bool)
                          n207 = local write "send message"(w359) -> ()
                          n208 = local write "stop"(w362) -> ()
                        }
                      }
                    }
                    frame "MEAS_SIS_IV_SWEEP_TPD" {
                      n209 = stacked-sequence {
                        seq-local: [w376 _ _] -> [_ w399 _]
                        seq-local: [w373 _ _] -> [_ w396 _]
                        seq-local: [w375 _ _] -> [_ w395 _]
                        seq-local: [w374 _ _] -> [_ w397 _]
                        seq-local: [_ w398 _] -> [_ _ w450]
                        seq-local: [w366 _ _] -> [_ w394 _]
                        seq-local: [w365 _ _] -> [_ w393 _]
                        seq-local: [w364 _ _] -> [_ w392 _]
                        tunnel: w363 -> [_ _ w451]
                        frame #0 {
                          n210 = local read "option"() -> (w385:string)
                          n211 = Scan From String(format string="%d %d %f %f %f %s", input string=w385) -> (error out=w378:errorcluster, output 1=w374:i32, output 2=w373:i32, output 3=w375:dbl, output 4=w366:dbl, output 5=w365:dbl, output 6=w364:string)  [unwired: 8 in, 2 out]
                          n212 = case shown="에러" w378 {
                            tunnel: [TRUE FALSE] -> w377
                            frame No Error {
                            }
                            frame Error {
                            }
                          }
                          n213 = case shown="0, 1" w374 {
                            tunnel: [FALSE TRUE] -> w381
                            frame Default {
                            }
                            frame 0, 1 {
                            }
                          }
                          n214 = case shown="기본" w373 {
                            tunnel: [FALSE TRUE] -> w380
                            frame Default {
                            }
                            frame 1, 2 {
                            }
                          }
                          n215 = In Range and Coerce(upper limit=5.0, x=w365, lower limit=-5.0) -> (In Range?=w367:bool)  [unwired: 1 out]
                          n216 = In Range and Coerce(upper limit=20.0, x=w366, lower limit=-20.0) -> (In Range?=w368:bool)  [unwired: 1 out]
                          n217 = In Range and Coerce(upper limit=20.0, x=w375, lower limit=-20.0) -> (In Range?=w379:bool)  [unwired: 1 out]
                          n218 = Compound Arithmetic op=AND(w381, w380, w379, w377, w368, w367) -> (w376:bool)
                        }
                        frame #1 {
                          n219 = case shown="참" w399 {
                            tunnel: ["command error\n\rMRAS_SIS_IV_SWEEP pol(0 or 1) sb(1 or 2) start(-20 to 20) stop(-20 to 20) step(-5 to 5) \n\r" w405] -> w398
                            tunnel: w397 -> [_ w410]
                            tunnel: w396 -> [_ w409]
                            tunnel: w395 -> [_ w408]
                            tunnel: w394 -> [_ w407]
                            tunnel: w393 -> [_ w406]
                            tunnel: w392 -> [_ w402]
                            frame False {
                            }
                            frame True {
                              n220 = flat-sequence {
                                tunnel: w410 -> [w427]
                                tunnel: w409 -> [w426]
                                tunnel: w408 -> [w425]
                                tunnel: w407 -> [w422]
                                tunnel: w406 -> [w421]
                                tunnel: [w415] -> w404
                                tunnel: [w414] -> w403
                                tunnel: w402 -> [w413]
                                tunnel: [w412] -> w401
                                tunnel: [w432] -> w405
                                tunnel: w404 -> [w437]
                                tunnel: w403 -> [w431]
                                tunnel: w401 -> [w430]
                                frame #0 {
                                w417 = 0.0
                                n221 = local read "SIScontrol"() -> (w418:u16)
                                n222 = local read "Control"() -> (w419:T2)
                                n223 = Bundle By Name(cluster=w419, "control"=w418, "Offset"=w417, "Set_SIS_volt"=w417, "GPIB_PM"=w413) -> (w416:T2)
                                n224 = local read "Bias_LO_equip"() -> (w428:T9)
                                n225 = Bundle By Name(cluster=w428, "POL"=w427, "sb"=w426) -> (w424:T9)
                                n226 = Bundle By Name(cluster="i-vクラスタ 2", "start(mV)"=w425, "stop(mV)"=w422, "step(mV)"=w421, "IF OFF/ON"=TRUE) -> (w420:T1)
                                n227 = local write "Bias_LO_equip"(w424) -> ()
                                n228 = local write "i-vクラスタ 2"(w420) -> ()
                                n229 = call "_get_iv_sweep3.vi"("i-vクラスタ"=w420, "Control"=w416, "Bias_LO_equip"=w424) -> ("Vset"=w414:dbl[], "VPデータクラスタ"=w412:cluster{"配列":dbl[], "配列 2":dbl[]}, "VIデータクラスタ"=w415:cluster{"配列":dbl[], "配列 2":dbl[]})  [unwired: 2 in]
                                }
                                frame #1 {
                                n230 = Unbundle(w430) -> ("配列 2"=w429:dbl[])  [unwired: 1 out]
                                n231 = Unbundle(w437) -> ("配列"=w434:dbl[], "配列 2"=w433:dbl[])
                                n232 = Array Size(array=w434) -> (size(s)=w436:i32)
                                n233 = for {
                                N: w436 -> [_]
                                shift-right: [w446] -> w432
                                shift-left: "" -> [w447]
                                tunnel: w434 -> [w449]
                                tunnel: w433 -> [w448]
                                tunnel: w431 -> [w443]
                                tunnel: w429 -> [w439]
                                i -> [w440]
                                n234 = Index Array(array=w443, index=w440) -> (element=w444:dbl)
                                n235 = Index Array(array=w448, index=w440) -> (element=w441:dbl)
                                n236 = Index Array(array=w449, index=w440) -> (element=w442:dbl)
                                n237 = Index Array(array=w439, index=w440) -> (element=w438:dbl)
                                n238 = Format Into String(format string="%f,%f,%f,%f\n\r", initial string=w447, w444, w442, w441, w438) -> (resulting string=w446:string)  [unwired: 1 in, 1 out]
                                }
                                }
                              }
                            }
                          }
                        }
                        frame #2 {
                          n239 = TCP Write(connection ID=w451, data in=w450) -> (error out=w452:errorcluster)  [unwired: 2 in, 2 out]
                          n240 = Unbundle By Name(w452) -> ("status"=w453:bool)
                          n241 = local write "send message"(w450) -> ()
                          n242 = local write "stop"(w453) -> ()
                        }
                      }
                    }
                    frame "SET_CLNA" {
                      n243 = stacked-sequence {
                        seq-local: [w462 _ _] -> [_ w521 _]
                        seq-local: [w476 _ _] -> [_ w520 _]
                        seq-local: [w460 _ _] -> [_ w517 _]
                        seq-local: [w475 _ _] -> [_ w519 _]
                        seq-local: [_ w518 _] -> [_ _ w547]
                        seq-local: [w459 _ _] -> [_ w516 _]
                        seq-local: [w458 _ _] -> [_ w515 _]
                        seq-local: [w457 _ _] -> [_ w514 _]
                        seq-local: [w456 _ _] -> [_ w513 _]
                        seq-local: [w455 _ _] -> [_ w512 _]
                        tunnel: w454 -> [_ _ w548]
                        frame #0 {
                          n244 = local read "option"() -> (w481:string)
                          n245 = Scan From String(format string="%d %d %f %f %f %f %f %f", input string=w481) -> (error out=w477:errorcluster, output 1=w475:i32, output 2=w476:i32, output 3=w463:dbl, output 4=w461:dbl, output 5=w474:dbl, output 6=w473:dbl, output 7=w472:dbl, output 8=w471:dbl)  [unwired: 10 in, 2 out]
                          n246 = stacked-sequence {
                            tunnel: w463 -> [w483 _ _]
                            tunnel: w461 -> [w482 _ _]
                            tunnel: w474 -> [_ w491 _]
                            tunnel: w473 -> [_ w490 _]
                            tunnel: w472 -> [_ _ w499]
                            tunnel: w471 -> [_ _ w498]
                            tunnel: [w485 _ _] -> w469
                            tunnel: [w484 _ _] -> w468
                            tunnel: [_ w493 _] -> w467
                            tunnel: [_ w492 _] -> w466
                            tunnel: [_ _ w501] -> w465
                            tunnel: [_ _ w500] -> w464
                            tunnel: [w483 _ _] -> w460
                            tunnel: [w482 _ _] -> w459
                            tunnel: [_ w491 _] -> w458
                            tunnel: [_ w490 _] -> w457
                            tunnel: [_ _ w499] -> w456
                            tunnel: [_ _ w498] -> w455
                            frame #0 {
                              n247 = In Range and Coerce(upper limit=20.0, x=w482, lower limit=0.0) -> (In Range?=w484:bool)  [unwired: 1 out]
                              n248 = In Range and Coerce(upper limit=3.0, x=w483, lower limit=0.0) -> (In Range?=w485:bool)  [unwired: 1 out]
                            }
                            frame #1 {
                              n249 = In Range and Coerce(upper limit=20.0, x=w490, lower limit=0.0) -> (In Range?=w492:bool)  [unwired: 1 out]
                              n250 = In Range and Coerce(upper limit=3.0, x=w491, lower limit=0.0) -> (In Range?=w493:bool)  [unwired: 1 out]
                            }
                            frame #2 {
                              n251 = In Range and Coerce(upper limit=20.0, x=w498, lower limit=0.0) -> (In Range?=w500:bool)  [unwired: 1 out]
                              n252 = In Range and Coerce(upper limit=3.0, x=w499, lower limit=0.0) -> (In Range?=w501:bool)  [unwired: 1 out]
                            }
                          }
                          n253 = case shown="기본" w476 {
                            tunnel: [FALSE TRUE] -> w478
                            frame Default {
                            }
                            frame 1, 2 {
                            }
                          }
                          n254 = case shown="0, 1" w475 {
                            tunnel: [FALSE TRUE] -> w479
                            frame Default {
                            }
                            frame 0, 1 {
                            }
                          }
                          n255 = case shown="에러" w477 {
                            tunnel: [TRUE FALSE] -> w470
                            frame No Error {
                            }
                            frame Error {
                            }
                          }
                          n256 = Compound Arithmetic op=AND(w479, w478, w470, w469, w468, w467, w466, w465, w464) -> (w462:bool)
                        }
                        frame #1 {
                          n257 = case shown="참" w521 {
                            tunnel: w520 -> [_ w540]
                            tunnel: w519 -> [_ w541]
                            tunnel: ["command error\n\rSET_CLNA pol(0 or 1) sb(1 or 2) VD1(0 to 3) ID1(0 to 30) VD2 ID2 VD3 ID3 \n\r" w539] -> w518
                            tunnel: w517 -> [_ w531]
                            tunnel: w516 -> [_ w530]
                            tunnel: w515 -> [_ w529]
                            tunnel: w514 -> [_ w528]
                            tunnel: w513 -> [_ w527]
                            tunnel: w512 -> [_ w526]
                            frame False {
                            }
                            frame True {
                              n258 = local read "CLNA_SET"() -> (w532:T7)
                              n259 = Bundle By Name(cluster=w532, "CLNA State"=1, "SET POL0 LNA1 STAGE1 DRAIN V"=w531, "SET POL0 LNA1 STAGE1 DRAIN C"=w530, "SET POL0 LNA1 STAGE2 DRAIN V"=w529, "SET POL0 LNA1 STAGE2 DRAIN C"=w528, "SET POL0 LNA1 STAGE3 DRAIN V"=w527, "SET POL0 LNA1 STAGE3 DRAIN C"=w526) -> (w524:T7)
                              n260 = local write "CLNA_SET"(w524) -> ()
                              n261 = local read "Bias_LO_equip"() -> (w542:T9)
                              n262 = Bundle By Name(cluster=w542, "POL"=w541, "sb"=w540) -> (w538:T9)
                              n263 = Unbundle By Name(w538) -> ("Slave Node in"=w536:cluster{"Address":i16, "Serial Number":i8[]}, "ObjHandle out"=w535:u32, "Cartridge band"=w537:u32, "sb"=w534:u32, "POL"=w533:u32)
                              n264 = local write "Bias_LO_equip"(w538) -> ()
                              n265 = call "WCA_SET_CLNA.vi"("Cartridge Band"=w537, "Slave Node in"=w536, "ObjHandle in"=w535, "POL"=w533, "sb"=w534, "CLNA_SET"=w524) -> ("error out"=w523:errorcluster)  [unwired: 8 in, 1 out]
                              n266 = case shown="에러 없음" w523 {
                                selector: w523 -> [_ w545]
                                tunnel: ["OK\n\r" w544] -> w539
                                frame No Error {
                                }
                                frame Error {
                                n267 = call <vilib>:"General Error Handler.vi"("type of dialog (OK msg:1)"=0, "error in (no error)"=w545) -> ("message"=w544:string)  [unwired: 9 in, 4 out]
                                }
                              }
                            }
                          }
                        }
                        frame #2 {
                          n268 = TCP Write(connection ID=w548, data in=w547) -> (error out=w549:errorcluster)  [unwired: 2 in, 2 out]
                          n269 = Unbundle By Name(w549) -> ("status"=w550:bool)
                          n270 = local write "stop"(w550) -> ()
                          n271 = local write "send message"(w547) -> ()
                        }
                      }
                    }
                    frame "GET_CLNA" {
                      n272 = stacked-sequence {
                        seq-local: [w552 _ _] -> [_ w570 _]
                        seq-local: [w555 _ _] -> [_ w569 _]
                        seq-local: [w554 _ _] -> [_ w568 _]
                        seq-local: [_ w567 _] -> [_ _ w601]
                        tunnel: w551 -> [_ _ w602]
                        frame #0 {
                          n273 = local read "option"() -> (w560:string)
                          n274 = Scan From String(format string="%d %d", input string=w560) -> (error out=w556:errorcluster, output 1=w554:i32, output 2=w555:i32)  [unwired: 4 in, 2 out]
                          n275 = case shown="기본" w555 {
                            tunnel: [FALSE TRUE] -> w557
                            frame Default {
                            }
                            frame 1, 2 {
                            }
                          }
                          n276 = case shown="0, 1" w554 {
                            tunnel: [FALSE TRUE] -> w558
                            frame Default {
                            }
                            frame 0, 1 {
                            }
                          }
                          n277 = case shown="에러" w556 {
                            tunnel: [TRUE FALSE] -> w553
                            frame No Error {
                            }
                            frame Error {
                            }
                          }
                          n278 = Compound Arithmetic op=AND(w558, w557, w553) -> (w552:bool)
                        }
                        frame #1 {
                          n279 = case shown="참" w570 {
                            tunnel: w569 -> [_ w595]
                            tunnel: w568 -> [_ w592]
                            tunnel: ["command error\n\rGET_CLNA pol(0 or 1) sb(1 or 2) " w594] -> w567
                            frame False {
                            }
                            frame True {
                              n280 = local read "Bias_LO_equip"() -> (w596:T9)
                              n281 = Bundle By Name(cluster=w596, "POL"=w592, "sb"=w595) -> (w593:T9)
                              n282 = Unbundle By Name(w593) -> ("Slave Node in"=w591:cluster{"Address":i16, "Serial Number":i8[]}, "ObjHandle out"=w590:u32, "Cartridge band"=w589:u32, "sb"=w587:u32, "POL"=w588:u32, "WCA_avg"=w586:i32)
                              n283 = local write "Bias_LO_equip"(w593) -> ()
                              n284 = call "WCA_GET_CLNA.vi"("Cartridge Band"=w589, "Slave Node in"=w591, "ObjHandle in"=w590, "POL"=w588, "sb"=w587, "avg"=w586) -> ("CLNA_monitor"=w584:T8, "error out"=w585:errorcluster)  [unwired: 7 in, 1 out]
                              n285 = Unbundle By Name(w584) -> ("Pol0 LNA1 S1 Drain V [V]"=w582:sgl, "Pol0 LNA1 S1 Drain C [mA]"=w581:sgl, "Pol0 LNA1 S1 Gate V [V]"=w580:sgl, "Pol0 LNA1 S2 Drain V [V]"=w579:sgl, "Pol0 LNA1 S2 Drain C [mA]"=w578:sgl, "Pol0 LNA1 S2 Gate V [V]"=w577:sgl, "Pol0 LNA1 S3 Drain V [V]"=w576:sgl, "Pol0 LNA1 S3 Drain C [mA]"=w575:sgl, "Pol0 LNA1 S3 Gate V [V]"=w574:sgl, "Pol0 LNA1 State"=w573:enum16{"Disabled", "Enabled"})
                              n286 = local write "CLNA_monitor"(w584) -> ()
                              n287 = Format Into String(format string="%f,%f,%f,%f,%f,%f,%f,%f,%f,%d\n\r", w582, w581, w580, w579, w578, w577, w576, w575, w574, w573) -> (resulting string=w572:string)  [unwired: 2 in, 1 out]
                              n288 = case shown="에러 없음" w585 {
                                selector: w585 -> [_ w599]
                                tunnel: [w597 w598] -> w594
                                tunnel: w572 -> [w597 _]
                                frame No Error {
                                }
                                frame Error {
                                n289 = call <vilib>:"General Error Handler.vi"("type of dialog (OK msg:1)"=0, "error in (no error)"=w599) -> ("message"=w598:string)  [unwired: 9 in, 4 out]
                                }
                              }
                            }
                          }
                        }
                        frame #2 {
                          n290 = TCP Write(connection ID=w602, data in=w601) -> (error out=w603:errorcluster)  [unwired: 2 in, 2 out]
                          n291 = Unbundle By Name(w603) -> ("status"=w604:bool)
                          n292 = local write "stop"(w604) -> ()
                          n293 = local write "send message"(w601) -> ()
                        }
                      }
                    }
                    frame "GET_CLNA_ALL" {
                      n294 = stacked-sequence {
                        seq-local: [w607 _] -> [_ w644]
                        tunnel: w605 -> [_ w645]
                        frame #0 {
                          n295 = for {
                            N: 2 -> [_]
                            shift-right: [w611] -> w607
                            shift-left: "" -> [w612]
                            i -> [w609]
                            n296 = for {
                              N: 2 -> [_]
                              shift-right: [w616] -> w611
                              shift-left: w612 -> [w617]
                              tunnel: w609 -> [w613]
                              i -> [w615]
                              n297 = local read "Bias_LO_equip"() -> (w639:T9)
                              n298 = Increment(x=w615) -> (x+1=w614:i32)
                              n299 = Bundle By Name(cluster=w639, "POL"=w613, "sb"=w614) -> (w638:T9)
                              n300 = Unbundle By Name(w638) -> ("Slave Node in"=w637:cluster{"Address":i16, "Serial Number":i8[]}, "ObjHandle out"=w636:u32, "Cartridge band"=w635:u32, "sb"=w633:u32, "POL"=w634:u32, "WCA_avg"=w632:i32)
                              n301 = local write "Bias_LO_equip"(w638) -> ()
                              n302 = call "WCA_GET_CLNA.vi"("Cartridge Band"=w635, "Slave Node in"=w637, "ObjHandle in"=w636, "POL"=w634, "sb"=w633, "avg"=w632) -> ("CLNA_monitor"=w630:T8, "error out"=w631:errorcluster)  [unwired: 7 in, 1 out]
                              n303 = Unbundle By Name(w630) -> ("Pol0 LNA1 S1 Drain V [V]"=w628:sgl, "Pol0 LNA1 S1 Drain C [mA]"=w627:sgl, "Pol0 LNA1 S1 Gate V [V]"=w626:sgl, "Pol0 LNA1 S2 Drain V [V]"=w625:sgl, "Pol0 LNA1 S2 Drain C [mA]"=w624:sgl, "Pol0 LNA1 S2 Gate V [V]"=w623:sgl, "Pol0 LNA1 S3 Drain V [V]"=w622:sgl, "Pol0 LNA1 S3 Drain C [mA]"=w621:sgl, "Pol0 LNA1 S3 Gate V [V]"=w620:sgl, "Pol0 LNA1 State"=w619:enum16{"Disabled", "Enabled"})
                              n304 = local write "CLNA_monitor"(w630) -> ()
                              n305 = Format Into String(format string="%f,%f,%f,%f,%f,%f,%f,%f,%f,%d\n\r", initial string=w617, w628, w627, w626, w625, w624, w623, w622, w621, w620, w619) -> (resulting string=w618:string)  [unwired: 1 in, 1 out]
                              n306 = case shown="에러 없음" w631 {
                                selector: w631 -> [_ w642]
                                tunnel: [w640 w641] -> w616
                                tunnel: w618 -> [w640 _]
                                frame No Error {
                                }
                                frame Error {
                                n307 = call <vilib>:"General Error Handler.vi"("type of dialog (OK msg:1)"=0, "error in (no error)"=w642) -> ("message"=w641:string)  [unwired: 9 in, 4 out]
                                }
                              }
                            }
                          }
                        }
                        frame #1 {
                          n308 = TCP Write(connection ID=w645, data in=w644) -> (error out=w646:errorcluster)  [unwired: 2 in, 2 out]
                          n309 = Unbundle By Name(w646) -> ("status"=w647:bool)
                          n310 = local write "stop"(w647) -> ()
                          n311 = local write "send message"(w644) -> ()
                        }
                      }
                    }
                    frame "SET_CLNA_OFF" {
                      n312 = stacked-sequence {
                        seq-local: [w649 _ _] -> [_ w667 _]
                        seq-local: [w652 _ _] -> [_ w666 _]
                        seq-local: [w651 _ _] -> [_ w665 _]
                        seq-local: [_ w664 _] -> [_ _ w687]
                        tunnel: w648 -> [_ _ w688]
                        frame #0 {
                          n313 = local read "option"() -> (w657:string)
                          n314 = Scan From String(format string="%d %d", input string=w657) -> (error out=w653:errorcluster, output 1=w651:i32, output 2=w652:i32)  [unwired: 4 in, 2 out]
                          n315 = case shown="기본" w652 {
                            tunnel: [FALSE TRUE] -> w654
                            frame Default {
                            }
                            frame 1, 2 {
                            }
                          }
                          n316 = case shown="0, 1" w651 {
                            tunnel: [FALSE TRUE] -> w655
                            frame Default {
                            }
                            frame 0, 1 {
                            }
                          }
                          n317 = case shown="에러" w653 {
                            tunnel: [TRUE FALSE] -> w650
                            frame No Error {
                            }
                            frame Error {
                            }
                          }
                          n318 = Compound Arithmetic op=AND(w655, w654, w650) -> (w649:bool)
                        }
                        frame #1 {
                          n319 = case shown="참" w667 {
                            tunnel: w666 -> [_ w680]
                            tunnel: w665 -> [_ w681]
                            tunnel: ["command error\n\rSET_CLNA pol(0 or 1) sb(1 or 2) VD1(0 to 3) ID1(0 to 30) VD2 ID2 VD3 ID3 \n\r" w679] -> w664
                            frame False {
                            }
                            frame True {
                              n320 = local read "CLNA_SET"() -> (w672:T7)
                              n321 = Bundle By Name(cluster=w672, "CLNA State"=0) -> (w670:T7)
                              n322 = local write "CLNA_SET"(w670) -> ()
                              n323 = local read "Bias_LO_equip"() -> (w682:T9)
                              n324 = Bundle By Name(cluster=w682, "POL"=w681, "sb"=w680) -> (w678:T9)
                              n325 = Unbundle By Name(w678) -> ("Slave Node in"=w676:cluster{"Address":i16, "Serial Number":i8[]}, "ObjHandle out"=w675:u32, "Cartridge band"=w677:u32, "sb"=w674:u32, "POL"=w673:u32)
                              n326 = local write "Bias_LO_equip"(w678) -> ()
                              n327 = call "WCA_SET_CLNA.vi"("Cartridge Band"=w677, "Slave Node in"=w676, "ObjHandle in"=w675, "POL"=w673, "sb"=w674, "CLNA_SET"=w670) -> ("error out"=w669:errorcluster)  [unwired: 8 in, 1 out]
                              n328 = case shown="에러 없음" w669 {
                                selector: w669 -> [_ w685]
                                tunnel: ["OK\n\r" w684] -> w679
                                frame No Error {
                                }
                                frame Error {
                                n329 = call <vilib>:"General Error Handler.vi"("type of dialog (OK msg:1)"=0, "error in (no error)"=w685) -> ("message"=w684:string)  [unwired: 9 in, 4 out]
                                }
                              }
                            }
                          }
                        }
                        frame #2 {
                          n330 = TCP Write(connection ID=w688, data in=w687) -> (error out=w689:errorcluster)  [unwired: 2 in, 2 out]
                          n331 = Unbundle By Name(w689) -> ("status"=w690:bool)
                          n332 = local write "stop"(w690) -> ()
                          n333 = local write "send message"(w687) -> ()
                        }
                      }
                    }
                    frame "SET_MAG_C" {
                      n334 = stacked-sequence {
                        seq-local: [w695 _ _] -> [_ w715 _]
                        seq-local: [w692 _ _] -> [_ w712 _]
                        seq-local: [w694 _ _] -> [_ w711 _]
                        seq-local: [w693 _ _] -> [_ w713 _]
                        seq-local: [_ w714 _] -> [_ _ w723]
                        tunnel: w691 -> [_ _ w724]
                        frame #0 {
                          n335 = local read "option"() -> (w704:string)
                          n336 = Scan From String(format string="%d %d %f", input string=w704) -> (error out=w697:errorcluster, output 1=w693:i32, output 2=w692:i32, output 3=w694:dbl)  [unwired: 5 in, 2 out]
                          n337 = case shown="0, 1" w693 {
                            tunnel: [FALSE TRUE] -> w700
                            frame Default {
                            }
                            frame 0, 1 {
                            }
                          }
                          n338 = case shown="기본" w692 {
                            tunnel: [FALSE TRUE] -> w699
                            frame Default {
                            }
                            frame 1, 2 {
                            }
                          }
                          n339 = case shown="에러" w697 {
                            tunnel: [TRUE FALSE] -> w696
                            frame No Error {
                            }
                            frame Error {
                            }
                          }
                          n340 = In Range and Coerce(upper limit=200.0, x=w694, lower limit=-200.0) -> (In Range?=w698:bool)  [unwired: 1 out]
                          n341 = Compound Arithmetic op=AND(w700, w699, w698, w696) -> (w695:bool)
                        }
                        frame #1 {
                          n342 = case shown="거짓" w715 {
                            tunnel: ["command error\n\rSET_MAG_C pol(0 or 1) sb(1 or 2) C(-200 to 200) \n\r" "OK\n\r"] -> w714
                            tunnel: w713 -> [_ w720]
                            tunnel: w712 -> [_ w719]
                            tunnel: w711 -> [_ w717]
                            frame False {
                            }
                            frame True {
                              n343 = local read "Bias_LO_equip"() -> (w722:T9)
                              n344 = Bundle By Name(cluster=w722, "POL"=w720, "sb"=w719) -> (w718:T9)
                              n345 = local write "Bias_LO_equip"(w718) -> ()
                              n346 = call "__SIS_Mag_C_Set.vi"("Set_Mag_C"=w717, "Bias_LO_equip"=w718) -> ()  [unwired: 10 in]
                            }
                          }
                        }
                        frame #2 {
                          n347 = TCP Write(connection ID=w724, data in=w723) -> (error out=w725:errorcluster)  [unwired: 2 in, 2 out]
                          n348 = Unbundle By Name(w725) -> ("status"=w726:bool)
                          n349 = local write "send message"(w723) -> ()
                          n350 = local write "stop"(w726) -> ()
                        }
                      }
                    }
                    frame "GET_MAG_VC" {
                      n351 = stacked-sequence {
                        seq-local: [w731 _ _] -> [_ w746 _]
                        seq-local: [w728 _ _] -> [_ w743 _]
                        seq-local: [w729 _ _] -> [_ w744 _]
                        seq-local: [_ w745 _] -> [_ _ w756]
                        tunnel: w727 -> [_ _ w757]
                        frame #0 {
                          n352 = local read "option"() -> (w736:string)
                          n353 = Scan From String(format string="%d %d", input string=w736) -> (error out=w732:errorcluster, output 1=w729:i32, output 2=w728:i32)  [unwired: 4 in, 2 out]
                          n354 = case shown="에러" w732 {
                            tunnel: [TRUE FALSE] -> w730
                            frame No Error {
                            }
                            frame Error {
                            }
                          }
                          n355 = case shown="0, 1" w729 {
                            tunnel: [FALSE TRUE] -> w734
                            frame Default {
                            }
                            frame 0, 1 {
                            }
                          }
                          n356 = case shown="기본" w728 {
                            tunnel: [FALSE TRUE] -> w733
                            frame Default {
                            }
                            frame 1, 2 {
                            }
                          }
                          n357 = Compound Arithmetic op=AND(w734, w733, w730) -> (w731:bool)
                        }
                        frame #1 {
                          n358 = case shown="거짓" w746 {
                            tunnel: ["command error\n\rGET_MAG_VC pol(0 or 1) sb(1 or 2)" w753] -> w745
                            tunnel: w744 -> [_ w752]
                            tunnel: w743 -> [_ w751]
                            frame False {
                            }
                            frame True {
                              n359 = local read "Bias_LO_equip"() -> (w755:T9)
                              n360 = Bundle By Name(cluster=w755, "POL"=w752, "sb"=w751) -> (w748:T9)
                              n361 = call "__SIS_Mag_Get.vi"("Bias_LO_equip"=w748) -> ("Get_Mag_I"=w749:dbl, "Get_Mag_V"=w750:dbl)  [unwired: 9 in]
                              n362 = local write "Bias_LO_equip"(w748) -> ()
                              n363 = Format Into String(format string="%f,%f\n\r", w750, w749) -> (resulting string=w753:string)  [unwired: 2 in, 1 out]
                            }
                          }
                        }
                        frame #2 {
                          n364 = TCP Write(connection ID=w757, data in=w756) -> (error out=w758:errorcluster)  [unwired: 2 in, 2 out]
                          n365 = Unbundle By Name(w758) -> ("status"=w759:bool)
                          n366 = local write "stop"(w759) -> ()
                          n367 = local write "send message"(w756) -> ()
                        }
                      }
                    }
                    frame "ACT_DEMAG" {
                      n368 = stacked-sequence {
                        seq-local: [w772 _ _] -> [_ w794 _]
                        seq-local: [w769 _ _] -> [_ w791 _]
                        seq-local: [w771 _ _] -> [_ w790 _]
                        seq-local: [w770 _ _] -> [_ w792 _]
                        seq-local: [_ w793 _] -> [_ _ w812]
                        seq-local: [w762 _ _] -> [_ w789 _]
                        seq-local: [w761 _ _] -> [_ w788 _]
                        tunnel: w760 -> [_ _ w813]
                        frame #0 {
                          n369 = local read "option"() -> (w781:string)
                          n370 = Scan From String(format string="%d %d %f %f %f", input string=w781) -> (error out=w774:errorcluster, output 1=w770:i32, output 2=w769:i32, output 3=w771:dbl, output 4=w762:dbl, output 5=w761:dbl)  [unwired: 7 in, 2 out]
                          n371 = case shown="에러" w774 {
                            tunnel: [TRUE FALSE] -> w773
                            frame No Error {
                            }
                            frame Error {
                            }
                          }
                          n372 = case shown="0, 1" w770 {
                            tunnel: [FALSE TRUE] -> w777
                            frame Default {
                            }
                            frame 0, 1 {
                            }
                          }
                          n373 = case shown="기본" w769 {
                            tunnel: [FALSE TRUE] -> w776
                            frame Default {
                            }
                            frame 1, 2 {
                            }
                          }
                          n374 = In Range and Coerce(upper limit=10000.0, x=w761, lower limit=0.0) -> (In Range?=w763:bool)  [unwired: 1 out]
                          n375 = In Range and Coerce(upper limit=100.0, x=w762, lower limit=0.0) -> (In Range?=w764:bool)  [unwired: 1 out]
                          n376 = In Range and Coerce(upper limit=200.0, x=w771, lower limit=0.0) -> (In Range?=w775:bool)  [unwired: 1 out]
                          n377 = Compound Arithmetic op=AND(w777, w776, w775, w773, w764, w763) -> (w772:bool)
                        }
                        frame #1 {
                          n378 = case shown="참" w794 {
                            tunnel: ["command error\n\rACT_DEMAG pol(0 or 1) sb(1 or 2) start(0 to 200) step(0 to 100) time(0 10000) \n\r" w796] -> w793
                            tunnel: w792 -> [_ w801]
                            tunnel: w791 -> [_ w800]
                            tunnel: w790 -> [_ w799]
                            tunnel: w789 -> [_ w798]
                            tunnel: w788 -> [_ w797]
                            frame False {
                            }
                            frame True {
                              n379 = flat-sequence {
                                tunnel: w801 -> [w809]
                                tunnel: w800 -> [w808]
                                tunnel: w799 -> [w802]
                                tunnel: w798 -> [w805]
                                tunnel: w797 -> [w804]
                                tunnel: ["OK\n\r"] -> w796
                                frame #0 {
                                n380 = local read "Bias_LO_equip"() -> (w810:T9)
                                n381 = Bundle By Name(cluster=w810, "POL"=w809, "sb"=w808) -> (w807:T9)
                                n382 = Bundle By Name(cluster="demag", "Start(mA)"=w802, "step"=w805, "Time(ms)"=w804) -> (w803:T3)
                                n383 = local write "Bias_LO_equip"(w807) -> ()
                                n384 = call "_Demagnetization.vi"("demag"=w803, "Bias_LO_equip"=w807) -> ()  [unwired: 10 in]
                                n385 = local write "demag"(w803) -> ()
                                }
                                frame #1 {
                                }
                              }
                            }
                          }
                        }
                        frame #2 {
                          n386 = TCP Write(connection ID=w813, data in=w812) -> (error out=w814:errorcluster)  [unwired: 2 in, 2 out]
                          n387 = Unbundle By Name(w814) -> ("status"=w815:bool)
                          n388 = local write "send message"(w812) -> ()
                          n389 = local write "stop"(w815) -> ()
                        }
                      }
                    }
                    frame "SET_PA_VD" {
                      n390 = stacked-sequence {
                        seq-local: [w819 _ _] -> [_ w835 _]
                        seq-local: [w818 _ _] -> [_ w832 _]
                        seq-local: [w817 _ _] -> [_ w833 _]
                        seq-local: [_ w834 _] -> [_ _ w854]
                        tunnel: w816 -> [_ _ w855]
                        frame #0 {
                          n391 = local read "option"() -> (w827:string)
                          n392 = Scan From String(format string="%d %f", input string=w827) -> (error out=w821:errorcluster, output 1=w817:i32, output 2=w818:dbl)  [unwired: 4 in, 2 out]
                          n393 = case shown="0, 1" w817 {
                            tunnel: [FALSE TRUE] -> w823
                            frame Default {
                            }
                            frame 0, 1 {
                            }
                          }
                          n394 = case shown="에러" w821 {
                            tunnel: [TRUE FALSE] -> w820
                            frame No Error {
                            }
                            frame Error {
                            }
                          }
                          n395 = In Range and Coerce(upper limit=2.5, x=w818, lower limit=0.0) -> (In Range?=w822:bool)  [unwired: 1 out]
                          n396 = Compound Arithmetic op=AND(w823, w822, w820) -> (w819:bool)
                        }
                        frame #1 {
                          n397 = case shown="거짓" w835 {
                            tunnel: ["command error\n\rSET_PA_VD pol(0 or 1) VD(0 to 2.5) \n\r" w846] -> w834
                            tunnel: w833 -> [_ w838]
                            tunnel: w832 -> [_ w840]
                            frame False {
                            }
                            frame True {
                              # "Band10 はPol0がPA-B\nPol1がPA-Aで逆転しているので"
                              n398 = case shown="0, 기본" w838 {
                                tunnel: [1 0] -> w837
                                frame 0, Default {
                                }
                                frame 1 {
                                }
                              }
                              n399 = local read "Bias_LO_equip"() -> (w847:T9)
                              n400 = Bundle By Name(cluster=w847, "POL"=w837) -> (w845:T9)
                              n401 = Unbundle By Name(w845) -> ("Slave Node in"=w844:cluster{"Address":i16, "Serial Number":i8[]}, "ObjHandle out"=w843:u32, "POL"=w841:u32, "Cartridge band"=w842:u32)
                              n402 = local write "Bias_LO_equip"(w845) -> ()
                              n403 = call "WCA_SET_PA_VD_band10.vi"("Cartridge Band"=w842, "Slave Node in"=w844, "ObjHandle in"=w843, "POL（P0、P1）"=w841, "SET_PA_VD"=w840) -> ("error out"=w839:errorcluster)  [unwired: 9 in, 1 out]
                              n404 = case shown="에러 없음" w839 {
                                selector: w839 -> [_ w852]
                                tunnel: ["OK\n\r" w851] -> w846
                                frame No Error {
                                }
                                frame Error {
                                n405 = call <vilib>:"General Error Handler.vi"("type of dialog (OK msg:1)"=0, "error in (no error)"=w852) -> ("message"=w851:string)  [unwired: 9 in, 4 out]
                                }
                              }
                              "SET_PA_VD" <- w840
                            }
                          }
                        }
                        frame #2 {
                          n406 = TCP Write(connection ID=w855, data in=w854) -> (error out=w856:errorcluster)  [unwired: 2 in, 2 out]
                          n407 = Unbundle By Name(w856) -> ("status"=w857:bool)
                          n408 = local write "send message"(w854) -> ()
                          n409 = local write "stop"(w857) -> ()
                        }
                      }
                    }
                    frame "SET_PA_VG" {
                      n410 = stacked-sequence {
                        seq-local: [w861 _ _] -> [_ w877 _]
                        seq-local: [w859 _ _] -> [_ w874 _]
                        seq-local: [w860 _ _] -> [_ w875 _]
                        seq-local: [_ w876 _] -> [_ _ w896]
                        tunnel: w858 -> [_ _ w897]
                        frame #0 {
                          n411 = local read "option"() -> (w869:string)
                          n412 = Scan From String(format string="%d %f", input string=w869) -> (error out=w863:errorcluster, output 1=w860:i32, output 2=w859:dbl)  [unwired: 4 in, 2 out]
                          n413 = case shown="0, 1" w860 {
                            tunnel: [FALSE TRUE] -> w865
                            frame Default {
                            }
                            frame 0, 1 {
                            }
                          }
                          n414 = case shown="에러" w863 {
                            tunnel: [TRUE FALSE] -> w862
                            frame No Error {
                            }
                            frame Error {
                            }
                          }
                          n415 = In Range and Coerce(upper limit=0.0, x=w859, lower limit=-2.0) -> (In Range?=w864:bool)  [unwired: 1 out]
                          n416 = Compound Arithmetic op=AND(w865, w864, w862) -> (w861:bool)
                        }
                        frame #1 {
                          n417 = case shown="거짓" w877 {
                            tunnel: ["command error\n\rSET_PA_VG pol(0 or 1) vg(-2 to 0) \n\r" w888] -> w876
                            tunnel: w875 -> [_ w880]
                            tunnel: w874 -> [_ w882]
                            frame False {
                            }
                            frame True {
                              # "Band10 はPol0がPA-B\nPol1がPA-Aで逆転しているので"
                              n418 = case shown="0, 기본" w880 {
                                tunnel: [1 0] -> w879
                                frame 0, Default {
                                }
                                frame 1 {
                                }
                              }
                              n419 = local read "Bias_LO_equip"() -> (w889:T9)
                              n420 = Bundle By Name(cluster=w889, "POL"=w879) -> (w887:T9)
                              n421 = Unbundle By Name(w887) -> ("Slave Node in"=w885:cluster{"Address":i16, "Serial Number":i8[]}, "ObjHandle out"=w886:u32, "POL"=w883:u32, "Cartridge band"=w884:u32)
                              n422 = local write "Bias_LO_equip"(w887) -> ()
                              n423 = call "WCA_SET_PA_VG_Band10.vi"("Cartridge Band"=w884, "Slave Node in"=w885, "ObjHandle in"=w886, "POL（P0、P1）"=w883, "SET_PA_VG"=w882) -> ("error out"=w881:errorcluster)  [unwired: 9 in, 1 out]
                              n424 = case shown="에러 없음" w881 {
                                selector: w881 -> [_ w894]
                                tunnel: ["OK\n\r" w893] -> w888
                                frame No Error {
                                }
                                frame Error {
                                n425 = call <vilib>:"General Error Handler.vi"("type of dialog (OK msg:1)"=0, "error in (no error)"=w894) -> ("message"=w893:string)  [unwired: 9 in, 4 out]
                                }
                              }
                              "SET_PA_VG" <- w882
                            }
                          }
                        }
                        frame #2 {
                          n426 = TCP Write(connection ID=w897, data in=w896) -> (error out=w898:errorcluster)  [unwired: 2 in, 2 out]
                          n427 = Unbundle By Name(w898) -> ("status"=w899:bool)
                          n428 = local write "stop"(w899) -> ()
                          n429 = local write "send message"(w896) -> ()
                        }
                      }
                    }
                    frame "GET_PA" {
                      n430 = stacked-sequence {
                        seq-local: [w901 _ _] -> [_ w914 _]
                        seq-local: [w903 _ _] -> [_ w913 _]
                        seq-local: [_ w912 _] -> [_ _ w946]
                        tunnel: w900 -> [_ _ w947]
                        frame #0 {
                          n431 = local read "option"() -> (w907:string)
                          n432 = Scan From String(format string="%d", input string=w907) -> (error out=w904:errorcluster, output 1=w903:i32)  [unwired: 3 in, 2 out]
                          n433 = case shown="0, 1" w903 {
                            tunnel: [FALSE TRUE] -> w905
                            frame Default {
                            }
                            frame 0, 1 {
                            }
                          }
                          n434 = case shown="에러" w904 {
                            tunnel: [TRUE FALSE] -> w902
                            frame No Error {
                            }
                            frame Error {
                            }
                          }
                          n435 = Compound Arithmetic op=AND(w905, w902) -> (w901:bool)
                        }
                        frame #1 {
                          n436 = case shown="참" w914 {
                            tunnel: w913 -> [_ w924]
                            tunnel: ["command error\n\rSET_CLNA pol(0 or 1) sb(1 or 2) VD1(0 to 3) ID1(0 to 30) VD2 ID2 VD3 ID3 \n\r" w930] -> w912
                            frame False {
                            }
                            frame True {
                              n437 = local read "Bias_LO_equip"() -> (w931:T9)
                              n438 = Bundle By Name(cluster=w931, "POL"=w924) -> (w929:T9)
                              n439 = Unbundle By Name(w929) -> ("Slave Node in"=w927:cluster{"Address":i16, "Serial Number":i8[]}, "ObjHandle out"=w926:u32, "Cartridge band"=w925:u32)  [unwired: 3 out]
                              n440 = local write "Bias_LO_equip"(w929) -> ()
                              n441 = call "WCA_GET_PA.vi"("Cartridge Band"=w925, "Slave Node in"=w927, "ObjHandle in"=w926) -> ("GET_PA"=w917:T6, "error out"=w916:errorcluster)  [unwired: 10 in, 1 out]
                              "GET_PA" <- w917
                              n442 = Unbundle By Name(w917) -> ("PA_A_DRAIN_V"=w923:sgl, "PA_A_DRAIN_C"=w922:sgl, "PA_A_GATE_V"=w921:sgl, "PA_B_DRAIN_V"=w920:sgl, "PA_B_DRAIN_C"=w919:sgl, "PA_B_GATE_V"=w918:sgl)
                              n443 = case shown="0, 기본" w924 {
                                tunnel: [w935 w940] -> w928
                                tunnel: w923 -> [_ w939]
                                tunnel: w922 -> [_ w938]
                                tunnel: w921 -> [_ w937]
                                tunnel: w920 -> [w934 _]
                                tunnel: w919 -> [w933 _]
                                tunnel: w918 -> [w932 _]
                                frame 1 {
                                n444 = Format Into String(format string="%f,%f,%f\n\r", w934, w933, w932) -> (resulting string=w935:string)  [unwired: 2 in, 1 out]
                                }
                                frame 0, Default {
                                n445 = Format Into String(format string="%f,%f,%f\n\r", w939, w938, w937) -> (resulting string=w940:string)  [unwired: 2 in, 1 out]
                                }
                              }
                              n446 = case shown="에러 없음" w916 {
                                selector: w916 -> [_ w944]
                                tunnel: [w942 w943] -> w930
                                tunnel: w928 -> [w942 _]
                                frame No Error {
                                }
                                frame Error {
                                n447 = call <vilib>:"General Error Handler.vi"("type of dialog (OK msg:1)"=0, "error in (no error)"=w944) -> ("message"=w943:string)  [unwired: 9 in, 4 out]
                                }
                              }
                            }
                          }
                        }
                        frame #2 {
                          n448 = TCP Write(connection ID=w947, data in=w946) -> (error out=w948:errorcluster)  [unwired: 2 in, 2 out]
                          n449 = Unbundle By Name(w948) -> ("status"=w949:bool)
                          n450 = local write "stop"(w949) -> ()
                          n451 = local write "send message"(w946) -> ()
                        }
                      }
                    }
                    frame "GET_WCA_LO" {
                      n452 = stacked-sequence {
                        seq-local: [w954 _] -> [_ w1005]
                        tunnel: w950 -> [_ w1006]
                        frame #0 {
                          n453 = stacked-sequence {
                            tunnel: "" -> [_ w990]
                            tunnel: [_ w965] -> w951
                            tunnel: [w955 _] -> w952
                            frame #0 {
                              n454 = local read "Bias_LO_equip"() -> (w956:T9)
                              n455 = Unbundle By Name(w956) -> ("Slave Node in"=w960:cluster{"Address":i16, "Serial Number":i8[]}, "ObjHandle out"=w959:u32, "Cartridge band"=w961:u32)
                              n456 = call "WCA_GET_PA.vi"("Cartridge Band"=w961, "Slave Node in"=w960, "ObjHandle in"=w959) -> ("GET_PA"=w957:T6, "error out"=w964:errorcluster)  [unwired: 10 in, 1 out]
                              n457 = local write "GET_PA"(w957) -> ()
                              n458 = call "WCA_GET_PLL.vi"("Cartridge Band"=w961, "Slave Node in"=w960, "ObjHandle in"=w959, "error in (no error)"=w964) -> ("GET_PLL"=→"GET_PLL":T5, "error out"=w962:errorcluster)  [unwired: 9 in, 1 out]
                              n459 = call "WCA_GET_AMC.vi"("Cartridge Band"=w961, "Slave Node in"=w960, "ObjHandle in"=w959, "error in (no error)"=w962) -> ("GET_AMC"=→"GET_AMC":T4, "error out"=w955:errorcluster)  [unwired: 9 in, 1 out]
                            }
                            frame #1 {
                              n460 = local read "GET_PA"() -> (w1000:T6)
                              n461 = Unbundle(w1000) -> ("PA_A_DRAIN_V"=w998:sgl, "PA_A_DRAIN_C"=w997:sgl, "PA_A_GATE_V"=w996:sgl, "PA_B_DRAIN_V"=w995:sgl, "PA_B_DRAIN_C"=w994:sgl, "PA_B_GATE_V"=w993:sgl, "PA_3V_SUPPLY_V"=w992:sgl, "PA_5V_MON"=w991:sgl)
                              n462 = Format Into String(format string="%f,%f,%f,\n\r%f,%f,%f,\n\r%f,%f,\n\r", initial string=w990, w998, w997, w996, w995, w994, w993, w992, w991) -> (resulting string=w981:string)  [unwired: 1 in, 1 out]
                              n463 = local read "GET_PLL"() -> (w989:T5)
                              n464 = Unbundle(w989) -> ("PLL_ASSY_T"=w987:sgl, "PLL_REF_TOT_P"=w986:sgl, "PLL_IF_TOT_P"=w985:sgl, "PLL_CORR_V"=w984:sgl, "PLL_LOCK_V"=w983:sgl, "PLL_5V_SUPPLY_V"=w982:sgl)  [unwired: 6 out]
                              n465 = Format Into String(format string="%f,%f,%f,%f,%f,%f,\\n\\r", initial string=w981, w987, w986, w985, w984, w983, w982) -> (resulting string=w978:string)  [unwired: 1 in, 1 out]
                              n466 = local read "GET_AMC"() -> (w980:T4)
                              n467 = Unbundle(w980) -> ("AMC_A_DRAIN_V"=w977:sgl, "AMC_A_DRAIN_C"=w976:sgl, "AMC_A_GATE_V"=w975:sgl, "AMC_B_DRAIN_V"=w974:sgl, "AMC_B_DRAIN_C"=w973:sgl, "AMC_B_GATE_V"=w972:sgl, "AMC_E_DRAIN_V"=w971:sgl, "AMC_E_DRAIN_C"=w970:sgl, "AMC_E_GATE_V"=w969:sgl, "AMC_3V_SUPPLY_V"=w968:sgl, "AMC_5V_MON"=w967:sgl, "AMC_MULT_D_V"=w966:sgl)
                              n468 = Format Into String(format string="%f,%f,%f,\n\r%f,%f,%f,\n\r%f,%f,%f,\n\r%f,%f,%f\n\r", initial string=w978, w977, w976, w975, w974, w973, w972, w971, w970, w969, w968, w967, w966) -> (resulting string=w965:string)  [unwired: 1 in, 1 out]
                            }
                          }
                          n469 = case shown="에러 없음" w952 {
                            selector: w952 -> [_ w1003]
                            tunnel: [w1001 w1002] -> w954
                            tunnel: w951 -> [w1001 _]
                            frame No Error {
                            }
                            frame Error {
                              n470 = call <vilib>:"General Error Handler.vi"("type of dialog (OK msg:1)"=0, "error in (no error)"=w1003) -> ("message"=w1002:string)  [unwired: 9 in, 4 out]
                            }
                          }
                        }
                        frame #1 {
                          n471 = TCP Write(connection ID=w1006, data in=w1005) -> (error out=w1007:errorcluster)  [unwired: 2 in, 2 out]
                          n472 = Unbundle By Name(w1007) -> ("status"=w1008:bool)
                          n473 = local write "stop"(w1008) -> ()
                          n474 = local write "send message"(w1005) -> ()
                        }
                      }
                    }
                    frame "GET_TEMP" {
                      n475 = stacked-sequence {
                        seq-local: [w1011 _ _] -> [_ w1023 _]
                        seq-local: [w1012 _ _] -> [_ w1022 _]
                        seq-local: [_ w1021 _] -> [_ _ w1033]
                        tunnel: w1009 -> [_ _ w1034]
                        frame #0 {
                          n476 = local read "option"() -> (w1016:string)
                          n477 = Scan From String(format string="%d", input string=w1016) -> (error out=w1013:errorcluster, output 1=w1012:i32)  [unwired: 3 in, 2 out]
                          n478 = case shown="0, 1" w1012 {
                            tunnel: [FALSE TRUE] -> w1014
                            frame Default {
                            }
                            frame 0, 1 {
                            }
                          }
                          n479 = case shown="에러" w1013 {
                            tunnel: [TRUE FALSE] -> w1010
                            frame No Error {
                            }
                            frame Error {
                            }
                          }
                          n480 = Compound Arithmetic op=AND(w1014, w1010) -> (w1011:bool)
                        }
                        frame #1 {
                          n481 = case shown="참" w1023 {
                            tunnel: w1022 -> [_ w1031]
                            tunnel: ["command error\n\rGET_TEMP pol(0 or 1)" w1029] -> w1021
                            frame False {
                            }
                            frame True {
                              n482 = local read "Bias_LO_equip"() -> (w1032:T9)
                              n483 = Bundle By Name(cluster=w1032, "POL"=w1031) -> (w1028:T9)
                              n484 = local write "Bias_LO_equip"(w1028) -> ()
                              n485 = call "__Temp_Get.vi"("Bias_LO_equip"=w1028) -> ("MixTemp"=w1025:dbl, "90/20K_temp"=w1026:dbl, "4K_Temp"=w1027:dbl)  [unwired: 8 in]
                              n486 = Format Into String(format string="%f,%f,%f\n\r", w1027, w1026, w1025) -> (resulting string=w1029:string)  [unwired: 2 in, 1 out]
                            }
                          }
                        }
                        frame #2 {
                          n487 = TCP Write(connection ID=w1034, data in=w1033) -> (error out=w1035:errorcluster)  [unwired: 2 in, 2 out]
                          n488 = Unbundle By Name(w1035) -> ("status"=w1036:bool)
                          n489 = local write "stop"(w1036) -> ()
                          n490 = local write "send message"(w1033) -> ()
                        }
                      }
                    }
                  }
                }
                frame Error {
                  w1042 = 56 items=["No Error", "Argument Error", "Memory Full", "Out of Zone", "End of File", "File Already Open", "Generic File IO Error", "File Not Found", "File Permission Error", "Disk Full", "Duplicate Path", "Too Many Files Open", "Not Enabled", "Resource File Not Found", "Cannot Add Resource", "Resource Not Found", "Image Not Found", "Image Memory Error", "Pen Does Not Exist", "Config Bad Type", "Config Token Not Found", "Config Parse Error", "Config Memory Error", "Bad External Code Format", "Bad External Code Offset", "External Code Not Present", "Null Window", "Destroy Window Mixup", "Null Menu", "Print Aborted", "Bad Print Record", "Print Driver Error", "Windows Error During Print", "Memory Error During Print", "Print Dialog Error", "Generic Print Error", "Invalid Device Refnum", "Device Not Found", "Device Parameter Error", "Device Unit Error", "Can't Open Device", "Device Call Aborted", "Generic Error", "Cancelled By User", "Object ID Too Low", "Object ID Too High", "Object Not In Heap", "Unknown Heap", "Bad DefProc ID", "DefProc Not In Table", "Message Out Of Range", "Null Method", "Unknown Message", "Manager Call Not Supported", "Bad address", "Connection In progress", "Connection timed out", "Connection is already in progress", "Network attribute not supported", "Network error", "Address in use", "System out of memory", "Connection aborted", "Connection refused", "Connection is not connected", "Connection is already connected", "Connection closed", "Initialize error (interapplication manager)", "Bad occurrence", "Wait on unbound occurrence handler", "Occurrence queue overflow", "Bad path", "Semaphore not signaled", "Unrecognized type (interapplication manager)"] ("2nd Error to Convert")
                  w1043 = 66 items=["No Error", "Argument Error", "Memory Full", "Out of Zone", "End of File", "File Already Open", "Generic File IO Error", "File Not Found", "File Permission Error", "Disk Full", "Duplicate Path", "Too Many Files Open", "Not Enabled", "Resource File Not Found", "Cannot Add Resource", "Resource Not Found", "Image Not Found", "Image Memory Error", "Pen Does Not Exist", "Config Bad Type", "Config Token Not Found", "Config Parse Error", "Config Memory Error", "Bad External Code Format", "Bad External Code Offset", "External Code Not Present", "Null Window", "Destroy Window Mixup", "Null Menu", "Print Aborted", "Bad Print Record", "Print Driver Error", "Windows Error During Print", "Memory Error During Print", "Print Dialog Error", "Generic Print Error", "Invalid Device Refnum", "Device Not Found", "Device Parameter Error", "Device Unit Error", "Can't Open Device", "Device Call Aborted", "Generic Error", "Cancelled By User", "Object ID Too Low", "Object ID Too High", "Object Not In Heap", "Unknown Heap", "Bad DefProc ID", "DefProc Not In Table", "Message Out Of Range", "Null Method", "Unknown Message", "Manager Call Not Supported", "Bad address", "Connection In progress", "Connection timed out", "Connection is already in progress", "Network attribute not supported", "Network error", "Address in use", "System out of memory", "Connection aborted", "Connection refused", "Connection is not connected", "Connection is already connected", "Connection closed", "Initialize error (interapplication manager)", "Bad occurrence", "Wait on unbound occurrence handler", "Occurrence queue overflow", "Bad path", "Semaphore not signaled", "Unrecognized type (interapplication manager)"] ("3rd Error to Convert")
                  w1044 = 64 items=["No Error", "Argument Error", "Memory Full", "Out of Zone", "End of File", "File Already Open", "Generic File IO Error", "File Not Found", "File Permission Error", "Disk Full", "Duplicate Path", "Too Many Files Open", "Not Enabled", "Resource File Not Found", "Cannot Add Resource", "Resource Not Found", "Image Not Found", "Image Memory Error", "Pen Does Not Exist", "Config Bad Type", "Config Token Not Found", "Config Parse Error", "Config Memory Error", "Bad External Code Format", "Bad External Code Offset", "External Code Not Present", "Null Window", "Destroy Window Mixup", "Null Menu", "Print Aborted", "Bad Print Record", "Print Driver Error", "Windows Error During Print", "Memory Error During Print", "Print Dialog Error", "Generic Print Error", "Invalid Device Refnum", "Device Not Found", "Device Parameter Error", "Device Unit Error", "Can't Open Device", "Device Call Aborted", "Generic Error", "Cancelled By User", "Object ID Too Low", "Object ID Too High", "Object Not In Heap", "Unknown Heap", "Bad DefProc ID", "DefProc Not In Table", "Message Out Of Range", "Null Method", "Unknown Message", "Manager Call Not Supported", "Bad address", "Connection In progress", "Connection timed out", "Connection is already in progress", "Network attribute not supported", "Network error", "Address in use", "System out of memory", "Connection aborted", "Connection refused", "Connection is not connected", "Connection is already connected", "Connection closed", "Initialize error (interapplication manager)", "Bad occurrence", "Wait on unbound occurrence handler", "Occurrence queue overflow", "Bad path", "Semaphore not signaled", "Unrecognized type (interapplication manager)"] ("1st Error to Convert")
                  n491 = call <vilib>:"Error to Warning.vi"("1st Error to Convert"=w1044, "2nd Error to Convert"=w1042, "3rd Error to Convert"=w1043, "error in"=w1041) -> ("warning out"=w1040:errorcluster)  [unwired: 11 in]
                  n492 = local read "c ID"() -> (w1046:refnum<k5>)
                  n493 = TCP Close Connection(connection ID=w1046, error in (no error)=w1040) -> (error out=w1045:errorcluster)  [unwired: 1 in, 1 out]
                  n494 = local write "リモートアドレス"("") -> ()
                  n495 = local write "exit"(TRUE) -> ()
                  n496 = local write "リモートポート"(0) -> ()
                  n497 = local write "接続中"(FALSE) -> ()
                  n498 = call <vilib>:"Simple Error Handler.vi"("error in (no error)"=w1045) -> ()  [unwired: 4 in, 5 out]
                }
              }
            }
            frame #3 {
              n499 = local read "exit"() -> (w1048:bool)
            }
          }
        }
      }
      frame Error {
      }
    }
  }
  "command:" <- w1
  "send message" <- w1
  "option" <- w1
  "接続中" <- w5
  "リモートアドレス" <- ""
  "リモートポート" <- 0
  "接続回数" <- 0
